vi "PointGrey Grasshopper_Cam.vi"(0 "Operation":T2(ring), 1 "Camera-specific in":variant, 5 "Exposure time (s)":dbl, 7 "Save path":path, 9 "Capture mode":enum16{"Single frame", "Sequence"}(ring), 11 "Capture button":refnum<vi>, 12 "Image in":variant, 14 "Frames in sequence":u32) -> (3 "Camera-specific out":variant, 4 "Status":T1)   [LabVIEW 2018]
uses:
  <vilib>/userdefined/High Color/IMAQdx.ctl
  <vilib>/vision/Image Controls.llb/IMAQ Image.ctl
  <vilib>/vision/driver/IMAQdx.llb/IMAQdx Camera Control Mode.ctl
  <vilib>/vision/driver/IMAQdx.llb/IMAQdx Acquisition Mode.ctl
  <vilib>/Platform/TimedLoop/XDataNode/timing_clust.ctl
  <vilib>/Platform/TimedLoop/XDataNode/nitl_modes.ctl
  <vilib>/Platform/TimedLoop/XDataNode/wakeup.ctl
  <vilib>/vision/driver/IMAQdx.llb/IMAQdx Buffer Number Mode.ctl
  <vilib>/platform/TimedLoop/XDataNode/XDataNode.xnode
  <vilib>/vision/driver/NI_Vision_Acquisition_Software.lvlib
  <resource>/objmgr/imaqdx.rc
  <vilib>/Platform/TimedLoop/XDataNode/XDNodeRunTimeDep.lvlib
  <vilib>/vision/NI_Vision_Development_Module.lvlib
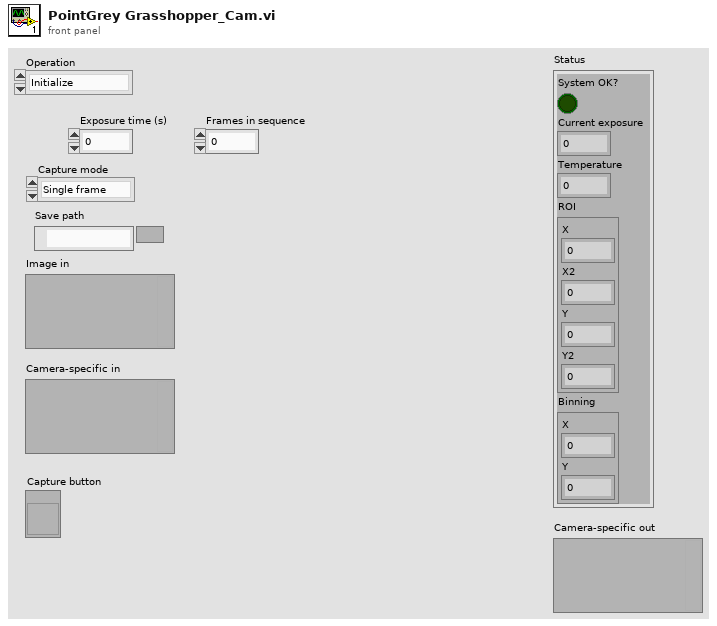
[diagram p1: front panel]
types:
  T1 = cluster{"System OK?":bool, "Current exposure":dbl, "Temperature":dbl, "ROI":cluster{"X":u32, "X2":u32, "Y":u32, "Y2":u32}, "Binning":cluster{"X":u32, "Y":u32}}
  T2 = enum16{"Initialize", "Shut down", "Set capture mode", "Set exposure", "Trigger and read", "Get status", "Other settings"}
  T3 = typedef "IMAQdx.ctl" = refnum<k21>
  T4 = typedef "IMAQ Image.ctl" = refnum<image>
  T5 = typedef "Semaphore RefNum" = refnum<k1>
  T6 = cluster{"Frames to capture":u32, "Current camera":i32, "Camera References":T3[], "Which cameras record":bool[], "Camera event refnums":refnum<event-registration>[], "Image buffers":T4[], "File write access":T5, "Offset and gain":dbl[][], "RGB Channels":enum16{"None", "Camera 1", "Camera 2", "Camera 3"}[], "RGB buffers":T4[], "Camera orientation":enum16{"No rotation, No flip", "No rotation, Flip UD", "No rotation, Flip LR", "Clockwise, No flip", "Clockwise, Flip UD", "Clockwise, Flip LR", "Anticlockwise, No flip", "Anticlockwise, Flip UD", "Anticlockwise, Flip LR"}[]}
  T7 = enum32{"Continuous", "Single frame", "Multi frame"}
  T8 = typedef "NI_Vision_Acquisition_Software.lvlib/IMAQdx Camera Control Mode.ctl" = enum32{"Controller", "Listener"}
  T9 = cluster{"New Image":T4, "Image":refnum<vi>, "FPS target":dbl}
  T10 = enum16{"open", "replace", "create", "open or create", "replace or create", "replace or create with confirmation"}
  T11 = cluster{"File refnum":refnum<file>, "Image File Directory":cluster{cluster{"Field":u16, "Type":u16, "Count":u32, "Value / Offset":u32, "Add IFD Offset?":bool}[], cluster{"Data":u32[], "Add offset?":bool}[]}, "Big endian?":bool, "IFD Offset Size":u32}
  T12 = typedef "NI_Vision_Acquisition_Software.lvlib/IMAQdx Acquisition Mode.ctl" = enum32{"One Shot", "Continuous"}
  T13 = typedef "XDNodeRunTimeDep.lvlib/timing_clust.ctl" = cluster{"Expected End [f-1]":u64, "Actual End [f-1]":u64, "Finished Late? [f-1]":bool, "Expected End [i-1]":u64, "Actual End [i-1]":u64, "Finished Late? [i-1]":bool, "Expected Start [i]":u64, "Actual Start [i]":u64, "Expected Start [f]":u64, "Actual Start [f]":u64, "Source Name":string, "Structure Name":string, "Period":i64, "Deadline":i64, "Offset":i64, "Start":i64, "Priority":i32, "Timeout":i32, "Mode":T14, "Wakeup Reason":T15, "Error":errorcluster, "Source Type":string, "Secondary Source Type":string, "Global End Time":u64, "Global Start Time":u64, "Frame Duration":u64, "Iteration Duration":u64, "Assigned CPU":i32, "I/O Scan Engine Mode":u32}
  T14 = typedef "XDNodeRunTimeDep.lvlib/nitl_modes.ctl" = enum32{"No Change", "Process missed periods, maintain original phase", "Discard missed periods, maintain original phase", "Process missed periods, ignore original phase", "Discard missed periods, ignore original phase"}
  T15 = typedef "XDNodeRunTimeDep.lvlib/wakeup.ctl" = enum32{"Normal", "Aborted", "Asynchronous wakeup", "Timing source error", "Timed loop error", "Timeout"}
  T16 = typedef "NI_Vision_Acquisition_Software.lvlib/IMAQdx Buffer Number Mode.ctl" = enum32{"Next", "Last", "Buffer Number", "Every", "Last New"}
  T17 = typedef "Image Type" = u32
  T18 = enum16{"No rotation, No flip", "No rotation, Flip UD", "No rotation, Flip LR", "Clockwise, No flip", "Clockwise, Flip UD", "Clockwise, Flip LR", "Anticlockwise, No flip", "Anticlockwise, Flip UD", "Anticlockwise, Flip LR"}[]
  T19 = enum16{"None", "Camera 1", "Camera 2", "Camera 3"}[]
  T20 = cluster{"Type":u32, "Version":u32, "Flags":u32, "SerialNumberHigh":u32, "SerialNumberLow":u32, "BusType":u32, "InterfaceName":string, "VendorName":string, "ModelName":string, "CameraFileName":string, "CameraAttributeURL":string}[]
  T21 = enum16{"None", "Camera 1", "Camera 2", "Camera 3"}
  T22 = cluster{"Camera identity":enum16{"Camera 1", "Camera 2", "Camera 3"}, "Timestamp":u64}
  T23 = enum16{"No rotation, No flip", "No rotation, Flip UD", "No rotation, Flip LR", "Clockwise, No flip", "Clockwise, Flip UD", "Clockwise, Flip LR", "Anticlockwise, No flip", "Anticlockwise, Flip UD", "Anticlockwise, Flip LR"}
  T24 = cluster{"element":enum16{"Camera 1", "Camera 2", "Camera 3"}, u64}
  T25 = cluster{"Camera identity":enum16{"Camera 1", "Camera 2", "Camera 3"}, "Timestamp":u64}[]
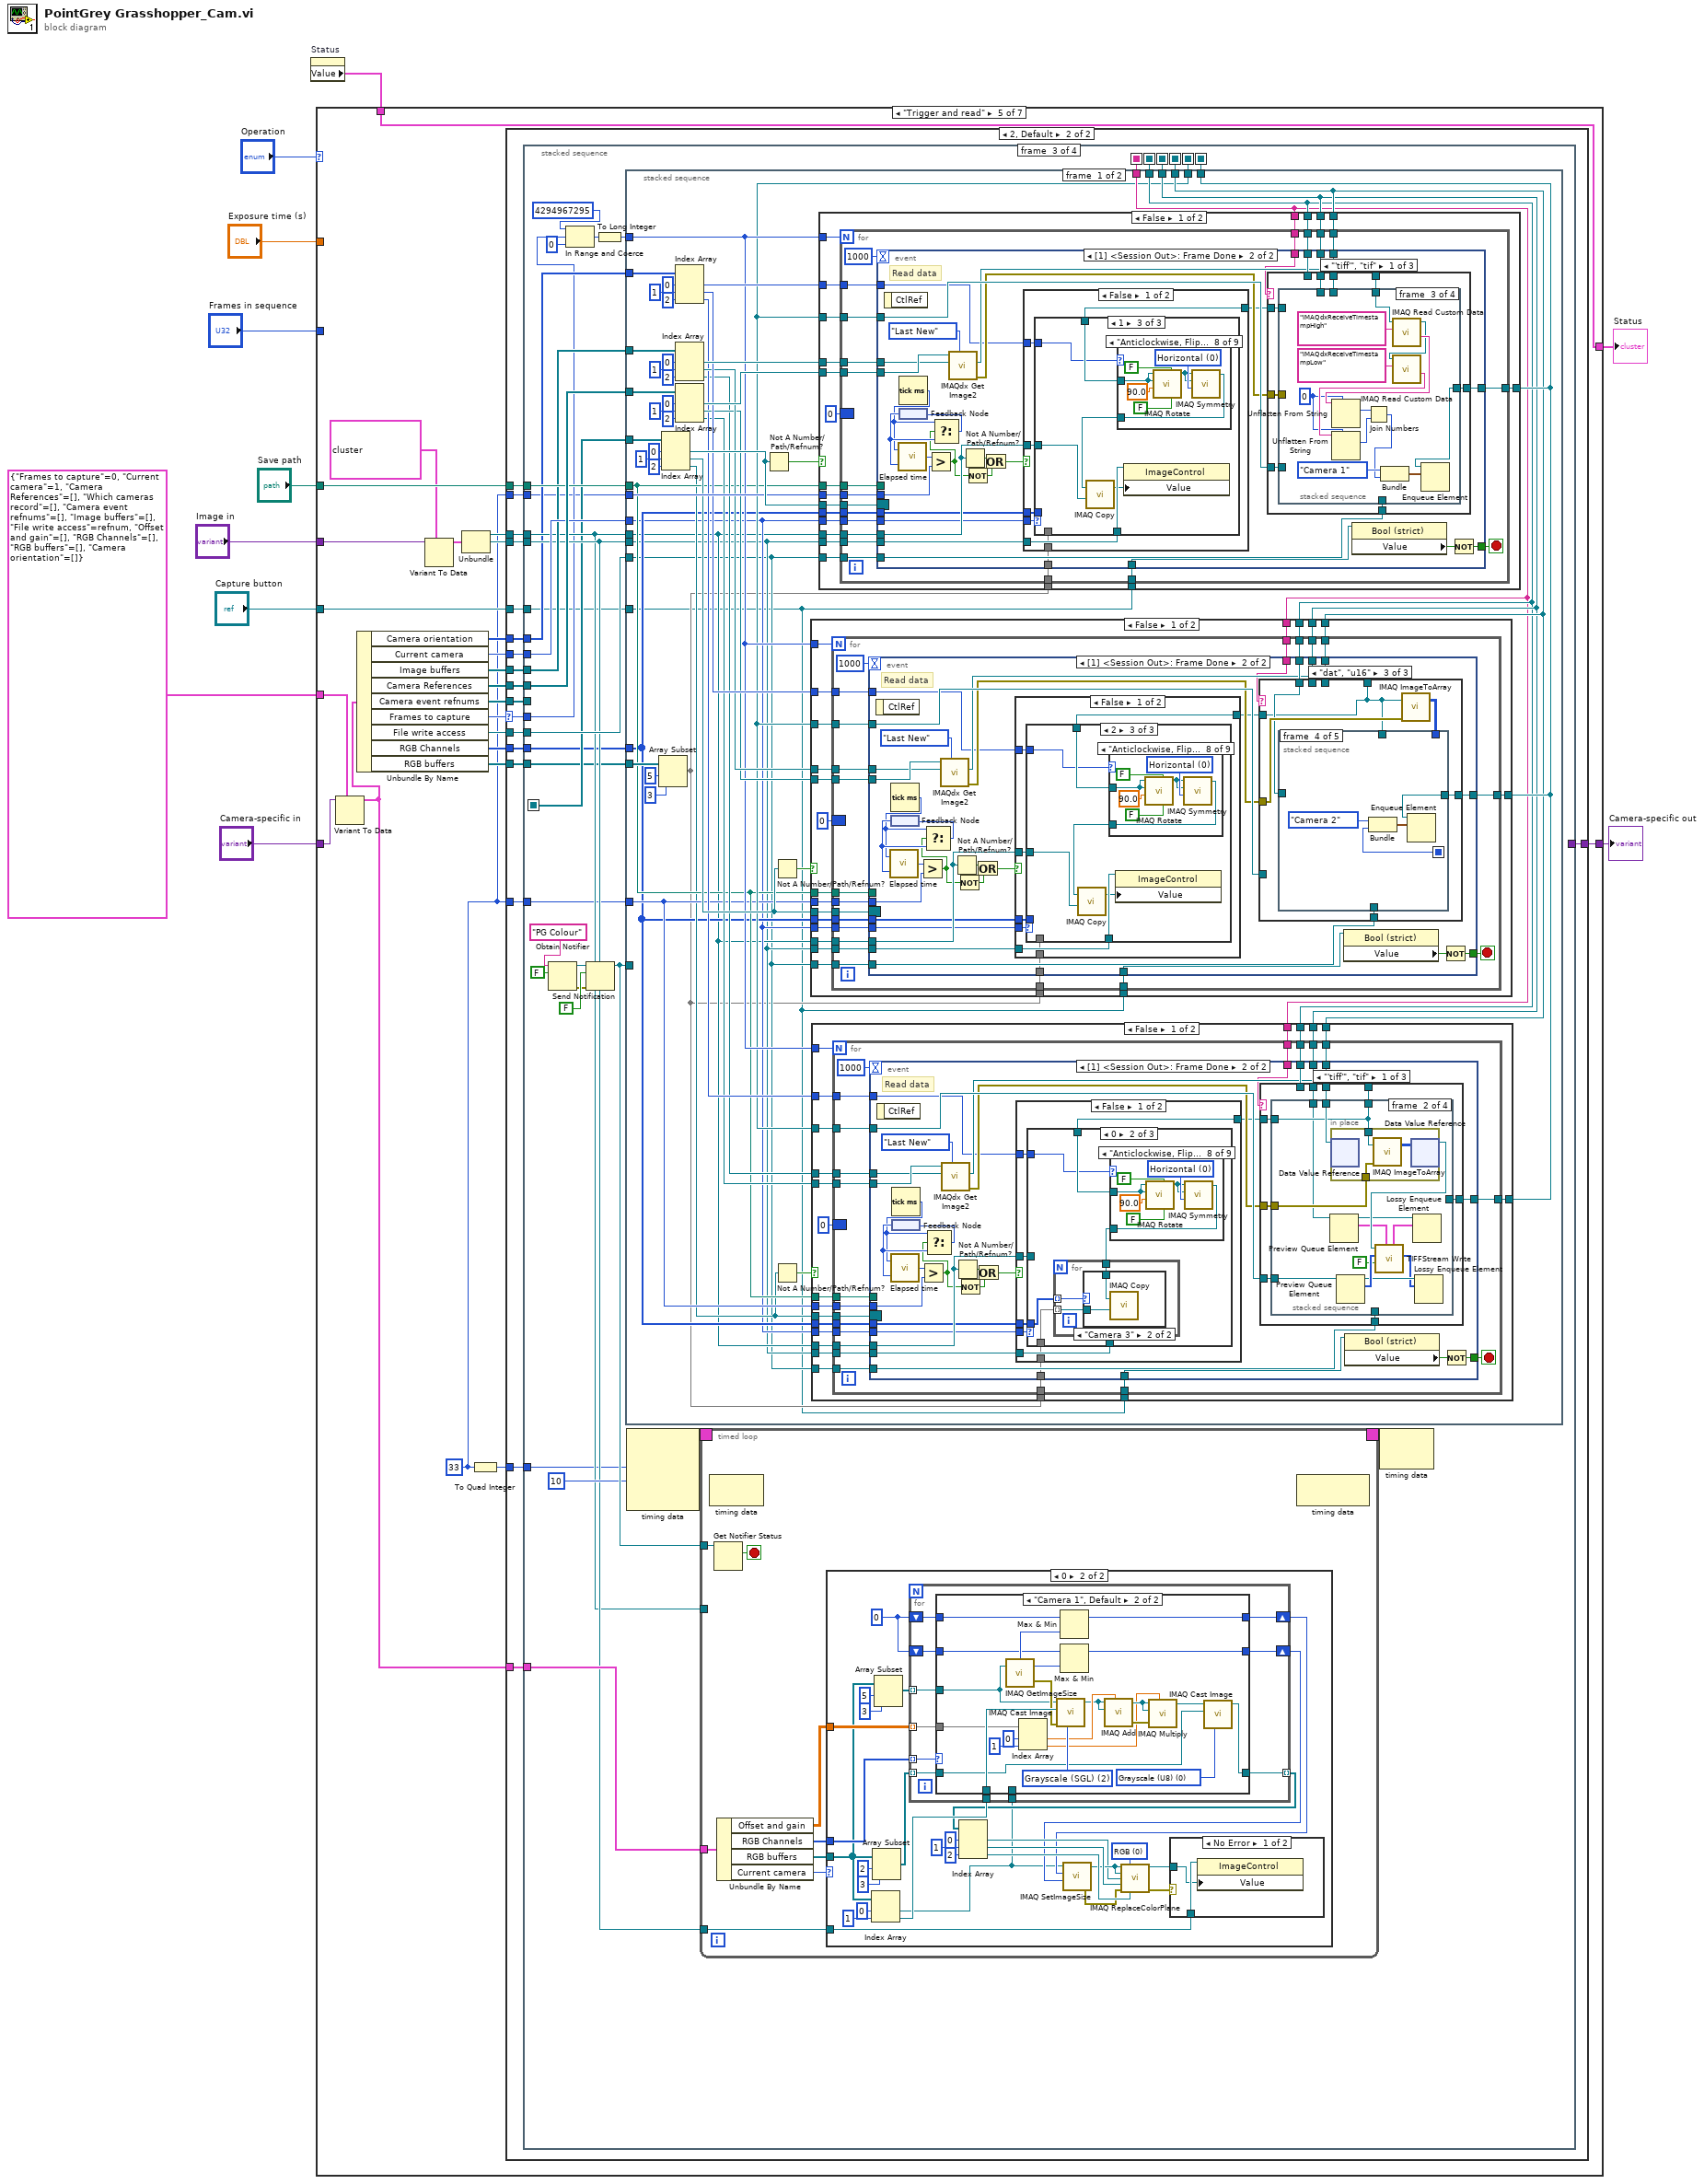
[diagram p0: block diagram]
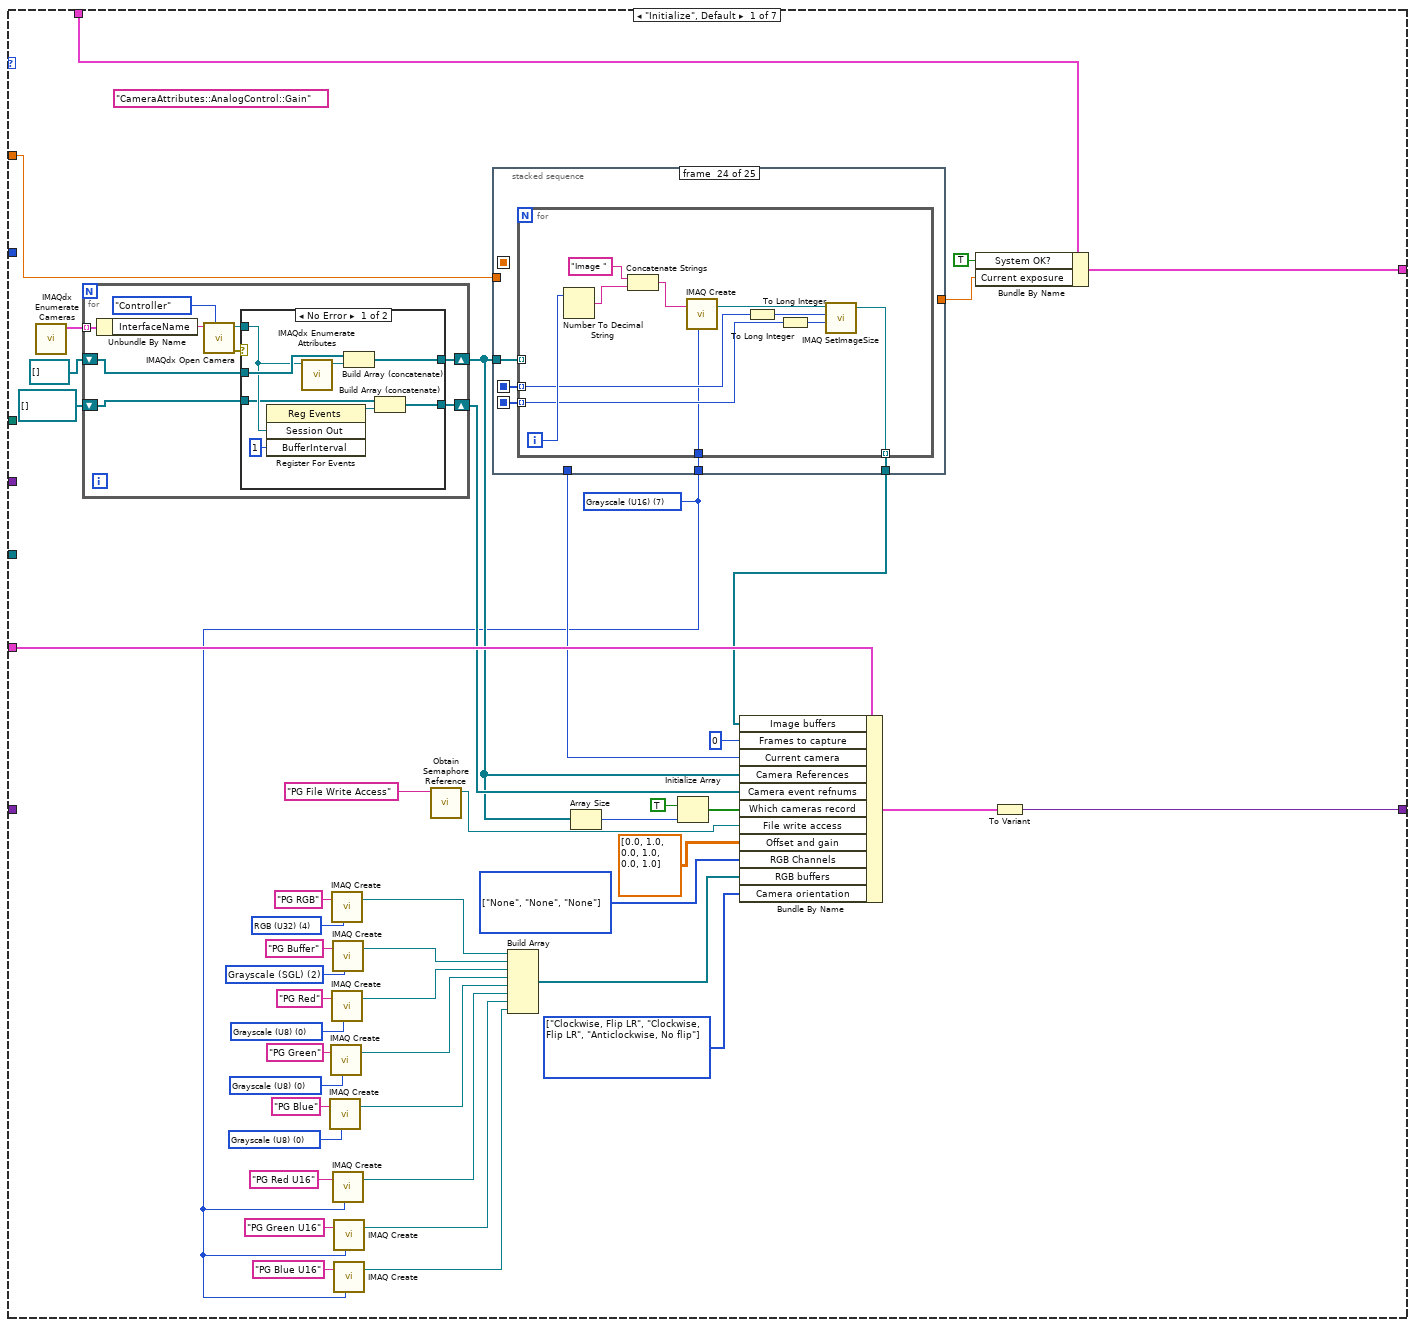
[diagram p2: hidden frame]
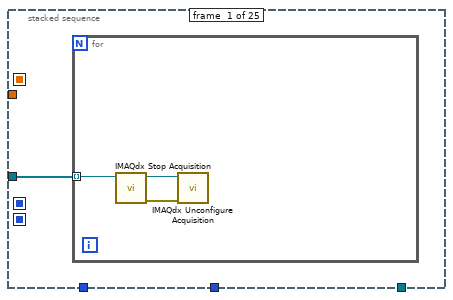
[diagram p3: hidden frame]
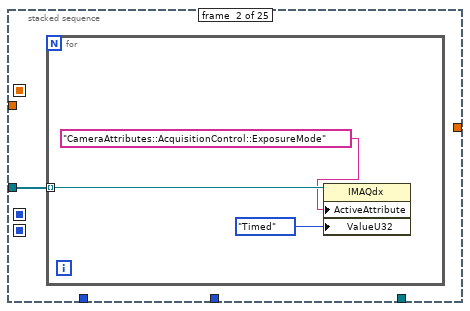
[diagram p4: hidden frame]
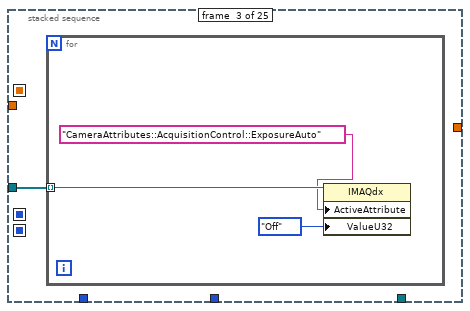
[diagram p5: hidden frame]
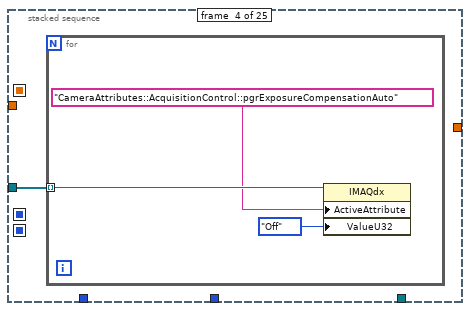
[diagram p6: hidden frame]
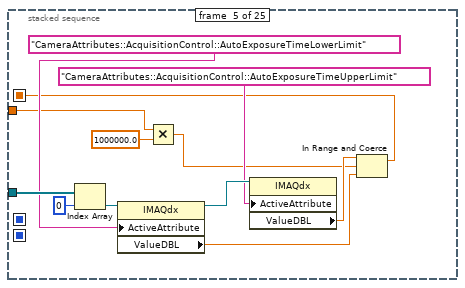
[diagram p7: hidden frame]
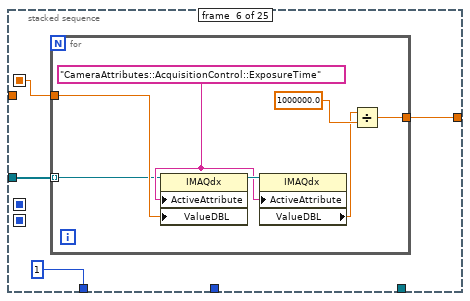
[diagram p8: hidden frame]
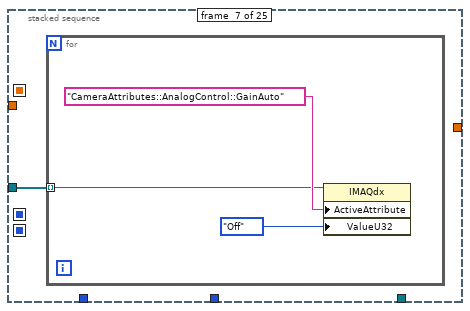
[diagram p9: hidden frame]
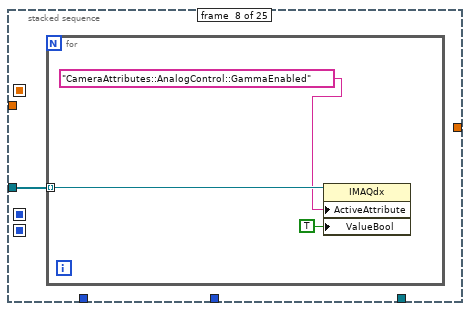
[diagram p10: hidden frame]
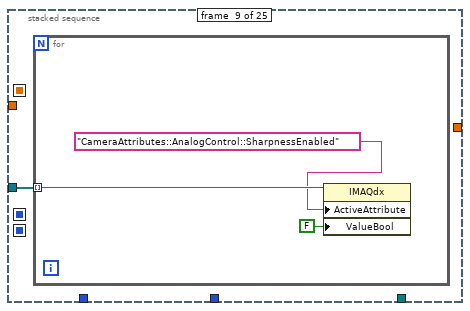
[diagram p11: hidden frame]
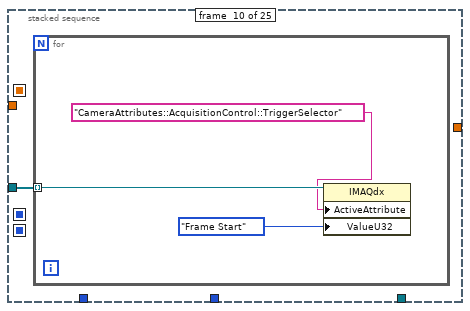
[diagram p12: hidden frame]
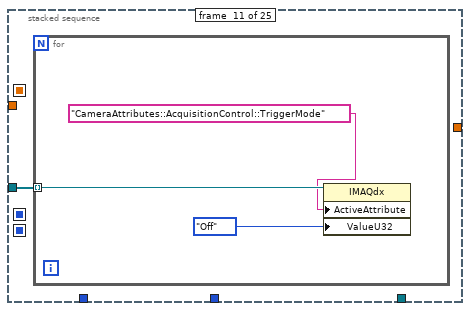
[diagram p13: hidden frame]
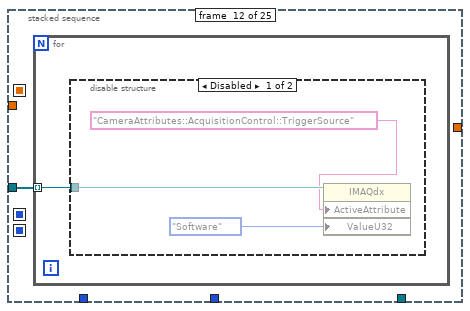
[diagram p14: hidden frame]
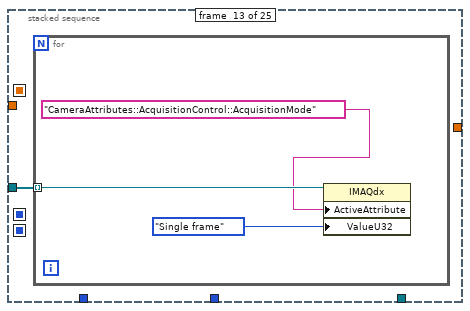
[diagram p16: hidden frame]
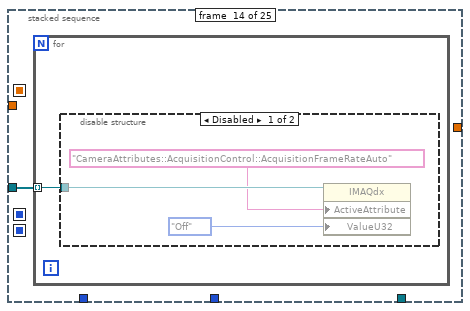
[diagram p17: hidden frame]
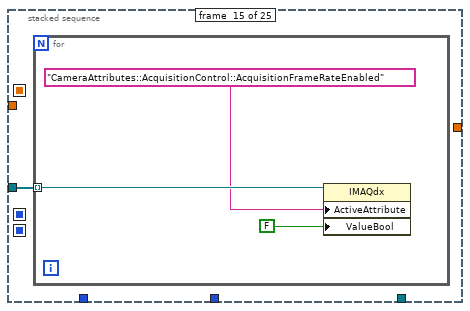
[diagram p19: hidden frame]
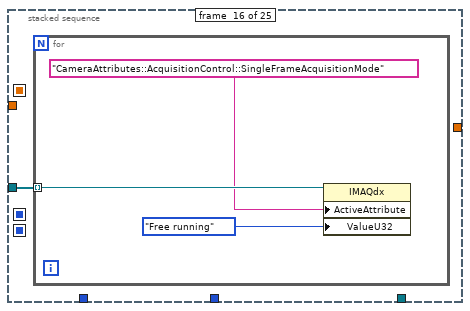
[diagram p20: hidden frame]
diagram:
  n1 = property on="Status" class="Clust (strict)"() -> ("Value"=w9:T1)  [unwired: 2 in, 2 out]
  n2 = case shown="\"Trigger and read\"" "Operation" {
    tunnel: "Exposure time (s)" -> [w47 _ _ w382 _ _ _]
    tunnel: w9 -> [w58 w218 w242 w388 w439 w1774 w1792]
    tunnel: [w57 w218 w242 w387 w439 w1773 w1792] -> w8
    tunnel: "Save path" -> [_ _ _ _ w438 _ _]
    tunnel: "Image in" -> [_ _ _ _ w429 _ _]
    tunnel: [w55 w213 w238 w385 w422 w1770 w1784] -> w5
    tunnel: "Camera-specific in" -> [_ w217 w240 w385 w425 w1770 w1791]
    tunnel: T6 {"Frames to capture"=0, "Current camera"=1, "Camera References"=[], "Which cameras record"=[], "Camera event refnums"=[], "Image buffers"=[], "File write access"=refnum, "Offset and gain"=[], "RGB Channels"=[], "RGB buffers"=[], "Camera orientation"=[]} -> [w56 w212 w239 w386 w437 w1769 w1790]
    tunnel: "Frames in sequence" -> [_ _ w235 _ _ _ _]
    tunnel: "Capture button" -> [_ _ _ _ w421 _ _]
    frame "Initialize", Default {
      w17 = T17 7 items=["Grayscale (U8)", "Grayscale (I16)", "Grayscale (SGL)", "Complex (CSG)", "RGB (U32)", "HSL (U32)", "RGB (U64)", "Grayscale (U16)"] ("Image Type")
      w19 = T18 [enum."Clockwise, Flip LR", enum."Clockwise, Flip LR", enum."Anticlockwise, No flip"] items=["No rotation, No flip", "No rotation, Flip UD", "No rotation, Flip LR", "Clockwise, No flip", "Clockwise, Flip UD", "Clockwise, Flip LR", "Anticlockwise, No flip", "Anticlockwise, Flip UD", "Anticlockwise, Flip LR"] ("Camera orientation")
      w26 = T17 0 items=["Grayscale (U8)", "Grayscale (I16)", "Grayscale (SGL)", "Complex (CSG)", "RGB (U32)", "HSL (U32)", "RGB (U64)", "Grayscale (U16)"] ("Image Type")
      w27 = T17 0 items=["Grayscale (U8)", "Grayscale (I16)", "Grayscale (SGL)", "Complex (CSG)", "RGB (U32)", "HSL (U32)", "RGB (U64)", "Grayscale (U16)"] ("Image Type")
      w28 = T17 0 items=["Grayscale (U8)", "Grayscale (I16)", "Grayscale (SGL)", "Complex (CSG)", "RGB (U32)", "HSL (U32)", "RGB (U64)", "Grayscale (U16)"] ("Image Type")
      w29 = T17 2 items=["Grayscale (U8)", "Grayscale (I16)", "Grayscale (SGL)", "Complex (CSG)", "RGB (U32)", "HSL (U32)", "RGB (U64)", "Grayscale (U16)"] ("Image Type")
      w30 = T17 4 items=["Grayscale (U8)", "Grayscale (I16)", "Grayscale (SGL)", "Complex (CSG)", "RGB (U32)", "HSL (U32)", "RGB (U64)", "Grayscale (U16)"] ("Image Type")
      w36 = T19 [enum."None", enum."None", enum."None"] items=["None", "Camera 1", "Camera 2", "Camera 3"] ("RGB Channels")
      (unwired) "CameraAttributes::AnalogControl::Gain"
      n3 = call <vilib>:"IMAQdx Enumerate Cameras.vi"() -> ("Camera Information Array"=w53:T20)  [unwired: 10 in, 1 out]
      n4 = for {
        tunnel: w53 -> [w198] mode=indexing
        shift-right: [w193] -> w45
        shift-left: T3[] [] -> [w191]
        shift-right: [w194] -> w50
        shift-left: refnum<event-registration>[] [] -> [w190]
        n5 = Unbundle By Name(w198) -> ("InterfaceName"=w197:string)
        n6 = call <vilib>:"IMAQdx Open Camera.vi"("Camera Control Mode"=IMAQdx_Camera_Control_Mode."Controller", "Session In"=w197) -> ("error out"=w192:errorcluster, "Session Out"=w195:T3)  [unwired: 8 in]
        n7 = case shown="No Error" w192 {
          tunnel: w195 -> [w202 _]
          tunnel: [w201 w207] -> w194
          tunnel: [w204 w208] -> w193
          tunnel: w191 -> [w203 w208]
          tunnel: w190 -> [w199 w207]
          frame No Error {
            n8 = register-events(w202, u32 1 ("BufferInterval")) -> (reference out=w200:refnum<event-registration>)  [unwired: 2 in, 1 out]
            n9 = call <vilib>:"IMAQdx Enumerate Attributes.vi"("Session In"=w202) -> ("Session Out"=w205:T3)  [unwired: 8 in, 2 out]
            n10 = Build Array (concatenate)(w203, w205) -> (w204:T3[])
            n11 = Build Array (concatenate)(w199, w200) -> (w201:refnum<event-registration>[])
          }
          frame Error {
          }
        }
      }
      n12 = call "IMAQ Create"("Image Name"="PG Blue", "Image Type"=w26) -> ("New Image"=w21:T4)  [unwired: 3 in, 1 out]
      n13 = call "IMAQ Create"("Image Name"="PG Green", "Image Type"=w27) -> ("New Image"=w22:T4)  [unwired: 3 in, 1 out]
      n14 = call "IMAQ Create"("Image Name"="PG RGB", "Image Type"=w30) -> ("New Image"=w25:T4)  [unwired: 3 in, 1 out]
      n15 = call "IMAQ Create"("Image Name"="PG Red", "Image Type"=w28) -> ("New Image"=w23:T4)  [unwired: 3 in, 1 out]
      n16 = call "IMAQ Create"("Image Name"="PG Buffer", "Image Type"=w29) -> ("New Image"=w24:T4)  [unwired: 3 in, 1 out]
      n17 = call "IMAQ Create"("Image Name"="PG Red U16", "Image Type"=w17) -> ("New Image"=w16:T4)  [unwired: 3 in, 1 out]
      n18 = call "IMAQ Create"("Image Name"="PG Green U16", "Image Type"=w17) -> ("New Image"=w14:T4)  [unwired: 3 in, 1 out]
      n19 = call "IMAQ Create"("Image Name"="PG Blue U16", "Image Type"=w17) -> ("New Image"=w15:T4)  [unwired: 3 in, 1 out]
      n20 = call <vilib>:"Obtain Semaphore Reference.vi"("name (unnamed)"="PG File Write Access") -> ("semaphore"=w38:T5)  [unwired: 4 in, 2 out]
      n21 = stacked-sequence {
        seq-local: [_ _ _ _ w78 _ _ _ _ _ _ _ _ _ _ _ _ _ _ _ _ _ _ _ _] -> [_ _ _ _ _ w87 _ _ _ _ _ _ _ _ _ _ _ _ _ _ _ _ _ _ _]
        seq-local: [_ _ _ _ _ _ _ _ _ _ _ _ _ _ _ _ _ w144 _ _ _ _ _ _ _] -> [_ _ _ _ _ _ _ _ _ _ _ _ _ _ _ _ _ _ _ _ _ _ _ w175 _]
        seq-local: [_ _ _ _ _ _ _ _ _ _ _ _ _ _ _ _ _ _ w150 _ _ _ _ _ _] -> [_ _ _ _ _ _ _ _ _ _ _ _ _ _ _ _ _ _ _ _ _ _ _ w174 _]
        tunnel: w45 -> [w59 w63 w67 w71 w84 w90 w98 w102 w106 w110 w114 w118 w123 w127 w132 w136 w140 w145 w151 w156 w160 w164 w168 w176 w188]
        tunnel: [_ _ _ _ _ 1 ("index") _ _ _ _ _ _ _ _ _ _ _ _ _ _ _ _ _ _ _] -> w48
        tunnel: w47 -> [_ _ _ _ w76 _ _ _ _ _ _ _ _ _ _ _ _ _ _ _ _ _ _ _ _]
        tunnel: [_ _ _ _ _ w88 _ _ _ _ _ _ _ _ _ _ _ _ _ _ _ _ _ _ _] -> w46
        tunnel: [_ _ _ _ _ _ _ _ _ _ _ _ _ _ _ _ _ _ _ _ _ _ _ w173 _] -> w41
        tunnel: w17 -> [_ _ _ _ _ _ _ _ _ _ _ _ _ _ _ _ _ _ _ _ _ _ _ w172 _]
        frame #0 {
          n22 = for {
            tunnel: w59 -> [w62] mode=indexing
            n23 = call <vilib>:"IMAQdx Stop Acquisition.vi"("Session In"=w62) -> ("error out"=w60:errorcluster, "Session Out"=w61:T3)  [unwired: 9 in]
            n24 = call <vilib>:"IMAQdx Unconfigure Acquisition.vi"("error in"=w60, "Session In"=w61) -> ()  [unwired: 8 in, 2 out]
          }
        }
        frame #1 {
          n25 = for {
            tunnel: w63 -> [w66] mode=indexing
            n26 = property class="IMAQdx"(reference=w66, "ActiveAttribute"="CameraAttributes::AcquisitionControl::ExposureMode", "ValueU32"=enum32{"Timed", "Trigger Width"}."Timed") -> ()  [unwired: 1 in, 2 out]
          }
        }
        frame #2 {
          n27 = for {
            tunnel: w67 -> [w70] mode=indexing
            n28 = property class="IMAQdx"(reference=w70, "ActiveAttribute"="CameraAttributes::AcquisitionControl::ExposureAuto", "ValueU32"=enum32{"Off", "Once", "Continuous"}."Off") -> ()  [unwired: 1 in, 2 out]
          }
        }
        frame #3 {
          n29 = for {
            tunnel: w71 -> [w74] mode=indexing
            n30 = property class="IMAQdx"(reference=w74, "ActiveAttribute"="CameraAttributes::AcquisitionControl::pgrExposureCompensationAuto", "ValueU32"=enum32{"Off", "Once", "Continuous"}."Off") -> ()  [unwired: 1 in, 2 out]
          }
        }
        frame #4 {
          n31 = Index Array(array=w84, index=0) -> (element=w86:T3)
          n32 = property class="IMAQdx"(reference=w86, "ActiveAttribute"="CameraAttributes::AcquisitionControl::AutoExposureTimeLowerLimit") -> (reference out=w82:T3, "ValueDBL"=w80:dbl)  [unwired: 1 in, 1 out]
          n33 = Multiply(x=w76, y=1000000.0) -> (x*y=w75:dbl)
          n34 = property class="IMAQdx"(reference=w82, "ActiveAttribute"="CameraAttributes::AcquisitionControl::AutoExposureTimeUpperLimit") -> ("ValueDBL"=w79:dbl)  [unwired: 1 in, 2 out]
          n35 = In Range and Coerce(upper limit=w79, x=w75, lower limit=w80) -> (coerced(x)=w78:dbl)  [unwired: 1 out]
        }
        frame #5 {
          n36 = for {
            tunnel: w90 -> [w91] mode=indexing
            tunnel: [w94] -> w88
            tunnel: w87 -> [w92]
            w93 = "CameraAttributes::AcquisitionControl::ExposureTime"
            n37 = property class="IMAQdx"(reference=w91, "ActiveAttribute"=w93, "ValueDBL"=w92) -> (reference out=w97:T3)  [unwired: 1 in, 1 out]
            n38 = property class="IMAQdx"(reference=w97, "ActiveAttribute"=w93) -> ("ValueDBL"=w95:dbl)  [unwired: 1 in, 2 out]
            n39 = Divide(x=w95, y=1000000.0) -> (x/y=w94:dbl)
          }
        }
        frame #6 {
          n40 = for {
            tunnel: w98 -> [w99] mode=indexing
            n41 = property class="IMAQdx"(reference=w99, "ActiveAttribute"="CameraAttributes::AnalogControl::GainAuto", "ValueU32"=enum32{"Off", "Once", "Continuous"}."Off") -> ()  [unwired: 1 in, 2 out]
          }
        }
        frame #7 {
          n42 = for {
            tunnel: w102 -> [w105] mode=indexing
            n43 = property class="IMAQdx"(reference=w105, "ActiveAttribute"="CameraAttributes::AnalogControl::GammaEnabled", "ValueBool"=TRUE) -> ()  [unwired: 1 in, 2 out]
          }
        }
        frame #8 {
          n44 = for {
            tunnel: w106 -> [w109] mode=indexing
            n45 = property class="IMAQdx"(reference=w109, "ActiveAttribute"="CameraAttributes::AnalogControl::SharpnessEnabled", "ValueBool"=FALSE) -> ()  [unwired: 1 in, 2 out]
          }
        }
        frame #9 {
          n46 = for {
            tunnel: w110 -> [w113] mode=indexing
            n47 = property class="IMAQdx"(reference=w113, "ActiveAttribute"="CameraAttributes::AcquisitionControl::TriggerSelector", "ValueU32"=enum32{"Frame Start", "Exposure Active"}."Frame Start") -> ()  [unwired: 1 in, 2 out]
          }
        }
        frame #10 {
          n48 = for {
            tunnel: w114 -> [w117] mode=indexing
            n49 = property class="IMAQdx"(reference=w117, "ActiveAttribute"="CameraAttributes::AcquisitionControl::TriggerMode", "ValueU32"=enum32{"Off", "On"}."Off") -> ()  [unwired: 1 in, 2 out]
          }
        }
        frame #11 {
          n50 = for {
            tunnel: w118 -> [w119] mode=indexing
            n51 = disable-structure shown="Disabled" {
              disable-tunnel: w119 -> [w122 _]
              frame Disabled {
                n52 = property class="IMAQdx"(reference=w122, "ActiveAttribute"="CameraAttributes::AcquisitionControl::TriggerSource", "ValueU32"=enum32{"Software", "Line 0", "Line 2", "Line 3"}."Software") -> ()  [unwired: 1 in, 2 out]
              }
              frame Enabled {
              }
            }
          }
        }
        frame #12 {
          n53 = for {
            tunnel: w123 -> [w126] mode=indexing
            n54 = property class="IMAQdx"(reference=w126, "ActiveAttribute"="CameraAttributes::AcquisitionControl::AcquisitionMode", "ValueU32"=T7."Single frame") -> ()  [unwired: 1 in, 2 out]
          }
        }
        frame #13 {
          n55 = for {
            tunnel: w127 -> [w128] mode=indexing
            n56 = disable-structure shown="Disabled" {
              disable-tunnel: w128 -> [w131 _]
              frame Disabled {
                n57 = property class="IMAQdx"(reference=w131, "ActiveAttribute"="CameraAttributes::AcquisitionControl::AcquisitionFrameRateAuto", "ValueU32"=enum32{"Off", "Continuous"}."Off") -> ()  [unwired: 1 in, 2 out]
              }
              frame Enabled {
              }
            }
          }
        }
        frame #14 {
          n58 = for {
            tunnel: w132 -> [w135] mode=indexing
            n59 = property class="IMAQdx"(reference=w135, "ActiveAttribute"="CameraAttributes::AcquisitionControl::AcquisitionFrameRateEnabled", "ValueBool"=FALSE) -> ()  [unwired: 1 in, 2 out]
          }
        }
        frame #15 {
          n60 = for {
            tunnel: w136 -> [w139] mode=indexing
            n61 = property class="IMAQdx"(reference=w139, "ActiveAttribute"="CameraAttributes::AcquisitionControl::SingleFrameAcquisitionMode", "ValueU32"=enum16{"Free running", "Triggered"}."Free running") -> ()  [unwired: 1 in, 2 out]
          }
        }
        frame #16 {
          n62 = for {
            tunnel: w140 -> [w143] mode=indexing
            w142 = u32 17563654 items=["Mono 8"=17301505, "Mono 12 Packed (IIDC-msb)"=17563654, "Mono 12 Packed"=17563719, "Mono 16"=17825799]
            n63 = property class="IMAQdx"(reference=w143, "ActiveAttribute"="CameraAttributes::ImageFormatControl::PixelFormat", "ValueU32"=w142) -> ()  [unwired: 1 in, 2 out]
          }
        }
        frame #17 {
          n64 = for {
            tunnel: w145 -> [w149] mode=indexing
            tunnel: [w146] -> w144 mode=indexing
            w148 = "CameraAttributes::ImageFormatControl::Width"
            n65 = property class="IMAQdx"(reference=w149, "ActiveAttribute"=w148) -> (reference out=w147:T3, "MaxU32"=w146:u32)  [unwired: 1 in, 1 out]
            n66 = property class="IMAQdx"(reference=w147, "ActiveAttribute"=w148, "ValueU32"=w146) -> ()  [unwired: 1 in, 2 out]
          }
        }
        frame #18 {
          n67 = for {
            tunnel: w151 -> [w155] mode=indexing
            tunnel: [w152] -> w150 mode=indexing
            w154 = "CameraAttributes::ImageFormatControl::Height"
            n68 = property class="IMAQdx"(reference=w155, "ActiveAttribute"=w154) -> (reference out=w153:T3, "MaxU32"=w152:u32)  [unwired: 1 in, 1 out]
            n69 = property class="IMAQdx"(reference=w153, "ActiveAttribute"=w154, "ValueU32"=w152) -> ()  [unwired: 1 in, 2 out]
          }
        }
        frame #19 {
          n70 = for {
            tunnel: w156 -> [w158] mode=indexing
            n71 = property class="IMAQdx"(reference=w158, "ActiveAttribute"="CameraAttributes::ImageFormatControl::OffsetX", "ValueU32"=u32 0) -> ()  [unwired: 1 in, 2 out]
          }
        }
        frame #20 {
          n72 = for {
            tunnel: w160 -> [w162] mode=indexing
            n73 = property class="IMAQdx"(reference=w162, "ActiveAttribute"="CameraAttributes::ImageFormatControl::OffsetY", "ValueU32"=u32 0) -> ()  [unwired: 1 in, 2 out]
          }
        }
        frame #21 {
          n74 = for {
            tunnel: w164 -> [w166] mode=indexing
            n75 = property class="IMAQdx"(reference=w166, "ActiveAttribute"="CameraAttributes::ImageFormatControl::BinningVertical", "ValueU32"=u32 1) -> ()  [unwired: 1 in, 2 out]
          }
        }
        frame #22 {
          n76 = for {
            tunnel: w168 -> [w170] mode=indexing
            w169 = u16 7 items=["Standard"=0, "2x2 Binning"=1, "2x2 Decimation"=2, "High sensitivity 12-bit ADC"=7]
            n77 = property class="IMAQdx"(reference=w170, "ActiveAttribute"="CameraAttributes::ImageFormatControl::VideoMode", "ValueU32"=w169) -> ()  [unwired: 1 in, 2 out]
          }
        }
        frame #23 {
          n78 = for {
            tunnel: w176 -> [_] mode=indexing
            tunnel: w175 -> [w181] mode=indexing
            tunnel: w174 -> [w180] mode=indexing
            tunnel: [w182] -> w173 mode=indexing
            tunnel: w172 -> [w177]
            i -> [w186]
            n79 = Number To Decimal String(number=w186) -> (decimal integer string=w185:string)  [unwired: 1 in]
            n80 = Concatenate Strings("Image ", w185) -> (w184:string)
            n81 = call "IMAQ Create"("Image Name"=w184, "Image Type"=w177) -> ("New Image"=w183:T4)  [unwired: 3 in, 1 out]
            n82 = To Long Integer(number=w181) -> (32bit integer=w179:i32)
            n83 = To Long Integer(number=w180) -> (32bit integer=w178:i32)
            n84 = call "IMAQ SetImageSize"("Y Resolution"=w178, "X Resolution"=w179, "Image"=w183) -> ("Image Out"=w182:T4)  [unwired: 2 in, 1 out]
          }
        }
        frame #24 {
          n85 = for {
            tunnel: w188 -> [w189] mode=indexing
            n86 = call <vilib>:"IMAQdx Configure Grab.vi"("Session In"=w189) -> ()  [unwired: 9 in, 2 out]
          }
        }
      }
      n87 = Build Array(w25, w24, w23, w22, w21, w16, w14, w15) -> (w20:T4[])
      n88 = Array Size(array=w45) -> (size(s)=w43:i32)
      n89 = Initialize Array(TRUE, w43) -> (w42:bool[])
      n90 = Bundle By Name(cluster=w56, "Image buffers"=w41, "Frames to capture"=u32 0, "Current camera"=w48, "Camera References"=w45, "Camera event refnums"=w50, "Which cameras record"=w42, "File write access"=w38, "Offset and gain"=dbl[][] [[0.0, 1.0], [0.0, 1.0], [0.0, 1.0]], "RGB Channels"=w36, "RGB buffers"=w20, "Camera orientation"=w19) -> (w51:T6)
      n91 = Bundle By Name(cluster=w58, "System OK?"=TRUE, "Current exposure"=w46) -> (w57:T1)
      n92 = To Variant(anything=w51) -> (Variant=w55:variant)
    }
    frame "Shut down" {
      n93 = Variant To Data(type=w212, Variant=w217) -> (data=w216:T6)  [unwired: 1 in, 1 out]
      n94 = Unbundle By Name(w216) -> ("Camera References"=w215:T3[], "Camera event refnums"=w214:refnum<event-registration>[], "File write access"=w211:T5, "Image buffers"=w210:T4[], "RGB buffers"=w209:T4[])
      n95 = for {
        tunnel: w210 -> [w220] mode=indexing
        n96 = call "IMAQ Dispose"("Image"=w220) -> ()  [unwired: 5 in, 1 out]
      }
      n97 = for {
        tunnel: w209 -> [w219] mode=indexing
        n98 = call "IMAQ Dispose"("Image"=w219) -> ()  [unwired: 5 in, 1 out]
      }
      n99 = stacked-sequence {
        tunnel: w215 -> [w221 _]
        tunnel: w214 -> [_ w227]
        frame #0 {
          n100 = for {
            tunnel: w221 -> [w222] mode=indexing
            n101 = call <vilib>:"IMAQdx Stop Acquisition.vi"("Session In"=w222) -> ("error out"=w226:errorcluster, "Session Out"=w225:T3)  [unwired: 9 in]
            n102 = call <vilib>:"IMAQdx Unconfigure Acquisition.vi"("error in"=w226, "Session In"=w225) -> ("error out"=w224:errorcluster, "Session Out"=w223:T3)  [unwired: 8 in]
            n103 = call <vilib>:"IMAQdx Close Camera.vi"("error in"=w224, "Session In"=w223) -> ()  [unwired: 9 in, 1 out]
          }
        }
        frame #1 {
          n104 = for {
            tunnel: w227 -> [w229] mode=indexing
            n105 = Unregister For Events(event registration refnum=w229) -> (error out=w228:errorcluster)  [unwired: 1 in]
            n106 = call <vilib>:"Clear Errors.vi"("error in (no error)"=w228) -> ()  [unwired: 5 in, 2 out]
          }
        }
      }
      n107 = call <vilib>:"Release Semaphore Reference.vi"("semaphore"=w211) -> ()  [unwired: 9 in, 2 out]
      n108 = To Variant(anything=w212) -> (Variant=w213:variant)
    }
    frame "Set capture mode" {
      n109 = Variant To Data(type=w239, Variant=w240) -> (data=w234:T6)  [unwired: 1 in, 1 out]
      n110 = Unbundle By Name(w234) -> ("Camera References"=w233:T3[], "Camera event refnums"=w231:refnum<event-registration>[], "Which cameras record"=w232:bool[])
      n111 = case shown="\"Sequence\"" "Capture mode" {
        tunnel: [w243 w313] -> w236
        tunnel: w235 -> [w244 w314]
        tunnel: w233 -> [w248 w318]
        tunnel: w232 -> [w247 w317]
        tunnel: w231 -> [w246 w316]
        tunnel: [w245 w315] -> w230
        frame "Sequence" {
          n112 = stacked-sequence {
            tunnel: w248 -> [_ w257]
            tunnel: w247 -> [_ w256]
            tunnel: w246 -> [w250 w253]
            tunnel: [_ w255] -> w245
            tunnel: w244 -> [w249 w254]
            tunnel: [w249 _] -> w243
            frame #0 {
              n113 = disable-structure shown="Enabled" {
                disable-tunnel: w250 -> [w251 _]
                frame Disabled {
                  n114 = for {
                    tunnel: w251 -> [w252] mode=indexing
                    n115 = Unregister For Events(event registration refnum=w252) -> ()  [unwired: 1 in, 1 out]
                  }
                }
                frame Enabled {
                }
              }
            }
            frame #1 {
              n116 = for {
                tunnel: w257 -> [w262] mode=indexing
                tunnel: w256 -> [w263] mode=indexing
                shift-right: [w261] -> w255
                shift-left: w253 -> [w260]
                tunnel: w254 -> [w259]
                i -> [w258]
                n117 = case shown="True" w263 {
                  tunnel: w262 -> [_ w267]
                  tunnel: [w264 w268] -> w261
                  tunnel: w260 -> [w264 w269]
                  tunnel: w259 -> [_ w266]
                  tunnel: w258 -> [_ w265]
                  frame False {
                  }
                  frame True {
                    n118 = stacked-sequence {
                      tunnel: w269 -> [_ _ _ _ _ _ _ _ w300 _]
                      tunnel: [_ _ _ _ _ _ _ _ w301 _] -> w268
                      tunnel: w267 -> [w272 w273 w281 w285 w288 w292 w294 w297 w302 w310]
                      tunnel: w266 -> [_ _ w280 _ _ _ _ _ _ _]
                      tunnel: w265 -> [_ _ _ _ _ _ _ _ w299 _]
                      frame #0 {
                        n119 = call <vilib>:"IMAQdx Stop Acquisition.vi"("Session In"=w272) -> ("error out"=w270:errorcluster, "Session Out"=w271:T3)  [unwired: 9 in]
                        n120 = call <vilib>:"IMAQdx Unconfigure Acquisition.vi"("error in"=w270, "Session In"=w271) -> ()  [unwired: 8 in, 2 out]
                      }
                      frame #1 {
                        n121 = disable-structure shown="Enabled" {
                          disable-tunnel: w273 -> [w274 w277]
                          frame Disabled {
                            n122 = property class="IMAQdx"(reference=w274, "ActiveAttribute"="CameraAttributes::AcquisitionControl::AcquisitionMode", "ValueU32"=T7."Multi frame") -> ()  [unwired: 1 in, 2 out]
                          }
                          frame Enabled {
                            n123 = property class="IMAQdx"(reference=w277, "ActiveAttribute"="CameraAttributes::AcquisitionControl::AcquisitionMode", "ValueU32"=T7."Continuous") -> ()  [unwired: 1 in, 2 out]
                          }
                        }
                      }
                      frame #2 {
                        n124 = disable-structure shown="Enabled" {
                          disable-tunnel: w281 -> [w283 _]
                          disable-tunnel: w280 -> [w282 _]
                          frame Disabled {
                            n125 = property class="IMAQdx"(reference=w283, "ActiveAttribute"="CameraAttributes::AcquisitionControl::AcquisitionFrameCount", "ValueU32"=w282) -> ()  [unwired: 1 in, 2 out]
                          }
                          frame Enabled {
                          }
                        }
                      }
                      frame #3 {
                        n126 = property class="IMAQdx"(reference=w285, "ActiveAttribute"="CameraAttributes::AcquisitionControl::TriggerSource", "ValueU32"=enum32{"Software", "Line 0", "Line 2", "Line 3"}."Software") -> ()  [unwired: 1 in, 2 out]
                      }
                      frame #4 {
                        n127 = property class="IMAQdx"(reference=w288, "ActiveAttribute"="CameraAttributes::AcquisitionControl::TriggerSelector", "ValueU32"=enum32{"Frame Start", "Exposure Active"}."Frame Start") -> ()  [unwired: 1 in, 2 out]
                      }
                      frame #5 {
                        n128 = property class="IMAQdx"(reference=w292, "ActiveAttribute"="CameraAttributes::AcquisitionControl::TriggerMode", "ValueU32"=enum32{"Off", "On"}."Off") -> ()  [unwired: 1 in, 2 out]
                      }
                      frame #6 {
                        n129 = property class="IMAQdx"(reference=w294, "ActiveAttribute"="CameraAttributes::AcquisitionControl::SingleFrameAcquisitionMode", "ValueU32"=enum16{"Free running", "Triggered"}."Triggered") -> ()  [unwired: 1 in, 2 out]
                      }
                      frame #7 {
                        n130 = disable-structure shown="Enabled" {
                          disable-tunnel: w297 -> [w298 _]
                          frame Disabled {
                            n131 = call <vilib>:"IMAQdx Configure Grab.vi"("Session In"=w298) -> ()  [unwired: 9 in, 2 out]
                          }
                          frame Enabled {
                          }
                        }
                      }
                      frame #8 {
                        n132 = disable-structure shown="Enabled" {
                          disable-tunnel: w302 -> [w308 _]
                          disable-tunnel: [w306 w309] -> w301
                          disable-tunnel: w300 -> [w305 w309]
                          disable-tunnel: w299 -> [w303 _]
                          frame Disabled {
                            n133 = register-events(w308, u32 1 ("BufferInterval")) -> (reference out=w304:refnum<event-registration>)  [unwired: 2 in, 1 out]
                            n134 = Replace Array Subset(array=w305, new element=w304, index=w303) -> (w306:refnum<event-registration>[])
                          }
                          frame Enabled {
                          }
                        }
                      }
                      frame #9 {
                        n135 = property class="IMAQdx"(reference=w310, "ActiveAttribute"="AcquisitionAttributes::ReceiveTimestampMode", "ValueU32"=enum16{"None", "Tick count", "System time"}."System time") -> ()  [unwired: 1 in, 2 out]
                      }
                    }
                  }
                }
              }
            }
          }
        }
        frame "Single frame", Default {
          n136 = stacked-sequence {
            tunnel: w318 -> [_ w327]
            tunnel: w317 -> [_ w326]
            tunnel: w316 -> [w320 w323]
            tunnel: [_ w325] -> w315
            tunnel: w314 -> [_ w324]
            tunnel: [u32 0 ("Frames in sequence") _] -> w313
            frame #0 {
              n137 = disable-structure shown="Enabled" {
                disable-tunnel: w320 -> [w321 _]
                frame Disabled {
                  n138 = for {
                    tunnel: w321 -> [w322] mode=indexing
                    n139 = Unregister For Events(event registration refnum=w322) -> ()  [unwired: 1 in, 1 out]
                  }
                }
                frame Enabled {
                }
              }
            }
            frame #1 {
              n140 = for {
                tunnel: w327 -> [w332] mode=indexing
                tunnel: w326 -> [w333] mode=indexing
                shift-right: [w331] -> w325
                shift-left: w323 -> [w330]
                tunnel: w324 -> [w329]
                i -> [w328]
                n141 = case shown="True" w333 {
                  tunnel: w332 -> [_ w337]
                  tunnel: [w334 w338] -> w331
                  tunnel: w330 -> [w334 w339]
                  tunnel: w329 -> [_ w336]
                  tunnel: w328 -> [_ w335]
                  frame False {
                  }
                  frame True {
                    n142 = stacked-sequence {
                      tunnel: w339 -> [_ w344 _ _ _ _ _ _ _]
                      tunnel: [_ w345 _ _ _ _ _ _ _] -> w338
                      tunnel: w337 -> [w342 w346 w354 w362 w366 w369 w373 w375 w378]
                      tunnel: w336 -> [_ _ _ w361 _ _ _ _ _]
                      tunnel: w335 -> [_ w343 _ _ _ _ _ _ _]
                      frame #0 {
                        n143 = call <vilib>:"IMAQdx Stop Acquisition.vi"("Session In"=w342) -> ("error out"=w340:errorcluster, "Session Out"=w341:T3)  [unwired: 9 in]
                        n144 = call <vilib>:"IMAQdx Unconfigure Acquisition.vi"("error in"=w340, "Session In"=w341) -> ()  [unwired: 8 in, 2 out]
                      }
                      frame #1 {
                        n145 = disable-structure shown="Enabled" {
                          disable-tunnel: w346 -> [w352 _]
                          disable-tunnel: [w350 w353] -> w345
                          disable-tunnel: w344 -> [w349 w353]
                          disable-tunnel: w343 -> [w347 _]
                          frame Disabled {
                            n146 = register-events(w352, u32 1 ("BufferInterval")) -> (reference out=w348:refnum<event-registration>)  [unwired: 2 in, 1 out]
                            n147 = Replace Array Subset(array=w349, new element=w348, index=w347) -> (w350:refnum<event-registration>[])
                          }
                          frame Enabled {
                          }
                        }
                      }
                      frame #2 {
                        n148 = disable-structure shown="Enabled" {
                          disable-tunnel: w354 -> [w355 w358]
                          frame Disabled {
                            n149 = property class="IMAQdx"(reference=w355, "ActiveAttribute"="CameraAttributes::AcquisitionControl::AcquisitionMode", "ValueU32"=T7."Multi frame") -> ()  [unwired: 1 in, 2 out]
                          }
                          frame Enabled {
                            n150 = property class="IMAQdx"(reference=w358, "ActiveAttribute"="CameraAttributes::AcquisitionControl::AcquisitionMode", "ValueU32"=T7."Continuous") -> ()  [unwired: 1 in, 2 out]
                          }
                        }
                      }
                      frame #3 {
                        n151 = disable-structure shown="Enabled" {
                          disable-tunnel: w362 -> [w364 _]
                          disable-tunnel: w361 -> [w363 _]
                          frame Disabled {
                            n152 = property class="IMAQdx"(reference=w364, "ActiveAttribute"="CameraAttributes::AcquisitionControl::AcquisitionFrameCount", "ValueU32"=w363) -> ()  [unwired: 1 in, 2 out]
                          }
                          frame Enabled {
                          }
                        }
                      }
                      frame #4 {
                        n153 = property class="IMAQdx"(reference=w366, "ActiveAttribute"="CameraAttributes::AcquisitionControl::TriggerSource", "ValueU32"=enum32{"Software", "Line 0", "Line 2", "Line 3"}."Software") -> ()  [unwired: 1 in, 2 out]
                      }
                      frame #5 {
                        n154 = property class="IMAQdx"(reference=w369, "ActiveAttribute"="CameraAttributes::AcquisitionControl::TriggerSelector", "ValueU32"=enum32{"Frame Start", "Exposure Active"}."Frame Start") -> ()  [unwired: 1 in, 2 out]
                      }
                      frame #6 {
                        n155 = property class="IMAQdx"(reference=w373, "ActiveAttribute"="CameraAttributes::AcquisitionControl::TriggerMode", "ValueU32"=enum32{"Off", "On"}."Off") -> ()  [unwired: 1 in, 2 out]
                      }
                      frame #7 {
                        n156 = property class="IMAQdx"(reference=w375, "ActiveAttribute"="CameraAttributes::AcquisitionControl::SingleFrameAcquisitionMode", "ValueU32"=enum16{"Free running", "Triggered"}."Triggered") -> ()  [unwired: 1 in, 2 out]
                      }
                      frame #8 {
                        n157 = disable-structure shown="Enabled" {
                          disable-tunnel: w378 -> [w379 _]
                          frame Disabled {
                            n158 = call <vilib>:"IMAQdx Configure Grab.vi"("Session In"=w379) -> ()  [unwired: 9 in, 2 out]
                          }
                          frame Enabled {
                          }
                        }
                      }
                    }
                  }
                }
              }
            }
          }
        }
      }
      n159 = Bundle By Name(cluster=w234, "Frames to capture"=w236, "Camera event refnums"=w230) -> (w237:T6)
      n160 = To Variant(anything=w237) -> (Variant=w238:variant)
    }
    frame "Set exposure" {
      n161 = Variant To Data(type=w386, Variant=w385) -> (data=w384:T6)  [unwired: 1 in, 1 out]
      n162 = Unbundle By Name(w384) -> ("Camera References"=w381:T3[], "Current camera"=w380:i32)
      n163 = case shown="1, Default" w380 {
        selector: w380 -> [_ w391]
        tunnel: [w389 w394] -> w383
        tunnel: w382 -> [w389 w393]
        tunnel: w381 -> [_ w392]
        frame 65535 {
        }
        frame 1, Default {
          n164 = Decrement(x=w391) -> (x-1=w390:i32)
          n165 = stacked-sequence {
            seq-local: [w399 _] -> [_ w408]
            tunnel: w392 -> [w405 w407]
            tunnel: w393 -> [w397 _]
            tunnel: [_ w409] -> w394
            tunnel: w390 -> [_ _]
            frame #0 {
              n166 = Index Array(array=w405, index=0) -> (element=w406:T3)
              n167 = property class="IMAQdx"(reference=w406, "ActiveAttribute"="CameraAttributes::AcquisitionControl::AutoExposureTimeLowerLimit") -> (reference out=w403:T3, "ValueDBL"=w401:dbl)  [unwired: 1 in, 1 out]
              n168 = Multiply(x=w397, y=1000000.0) -> (x*y=w396:dbl)
              n169 = property class="IMAQdx"(reference=w403, "ActiveAttribute"="CameraAttributes::AcquisitionControl::AutoExposureTimeUpperLimit") -> ("ValueDBL"=w400:dbl)  [unwired: 1 in, 2 out]
              n170 = In Range and Coerce(upper limit=w400, x=w396, lower limit=w401) -> (coerced(x)=w399:dbl)  [unwired: 1 out]
            }
            frame #1 {
              n171 = for {
                tunnel: [w413] -> w409
                tunnel: w408 -> [w411]
                tunnel: w407 -> [w410] mode=indexing
                w412 = "CameraAttributes::AcquisitionControl::ExposureTime"
                n172 = property class="IMAQdx"(reference=w410, "ActiveAttribute"=w412, "ValueDBL"=w411) -> (reference out=w416:T3)  [unwired: 1 in, 1 out]
                n173 = property class="IMAQdx"(reference=w416, "ActiveAttribute"=w412) -> ("ValueDBL"=w414:dbl)  [unwired: 1 in, 2 out]
                n174 = Divide(x=w414, y=1000000.0) -> (x/y=w413:dbl)
              }
            }
          }
        }
      }
      n175 = Bundle By Name(cluster=w388, "Current exposure"=w383) -> (w387:T1)
    }
    frame "Trigger and read" {
      w418 = u32 33 ("Period")
      n176 = Variant To Data(type=w437, Variant=w425) -> (data=w424:T6)  [unwired: 1 in, 1 out]
      n177 = Unbundle By Name(w424) -> ("Camera orientation"=w423:T18, "Current camera"=w432:i32, "Image buffers"=w433:T4[], "Camera References"=w435:T3[], "Camera event refnums"=w434:refnum<event-registration>[], "Frames to capture"=w436:u32, "File write access"=w426:T5, "RGB Channels"=w420:T19, "RGB buffers"=w419:T4[])
      n178 = Variant To Data(type=T9 {"New Image"=refnum, "Image"=refnum, "FPS target"=30.0} ("output cluster"), Variant=w429) -> (data=w431:T9)  [unwired: 1 in, 1 out]
      n179 = Unbundle(w431) -> ("New Image"=w428:T4, "Image"=w427:refnum<vi>)  [unwired: 1 out]
      n180 = To Quad Integer(1:w418) -> (0:w417:i64)
      n181 = case shown="2, Default" w436 {
        selector: w436 -> [_ w637]
        tunnel: w438 -> [w444 w643]
        tunnel: w428 -> [w445 w642]
        tunnel: w435 -> [w448 w641]
        tunnel: w434 -> [_ w640]
        tunnel: w433 -> [w447 w639]
        tunnel: w432 -> [w446 w638]
        tunnel: w427 -> [w443 w636]
        tunnel: w426 -> [_ w635]
        tunnel: w424 -> [w441 w634]
        tunnel: w423 -> [w442 w633]
        tunnel: [w440 w632] -> w422
        tunnel: w421 -> [_ w631]
        tunnel: w420 -> [_ w630]
        tunnel: w419 -> [_ w629]
        tunnel: w418 -> [_ w628]
        tunnel: w417 -> [_ w627]
        tunnel: w418 -> [_ w626]
        frame 0 {
          n182 = stacked-sequence {
            tunnel: w448 -> [w455 _]
            tunnel: w447 -> [w453 w547]
            tunnel: w446 -> [w452 _]
            tunnel: w445 -> [w451 w544]
            tunnel: w444 -> [w450 _]
            tunnel: w441 -> [_ w546]
            tunnel: w443 -> [_ w545]
            tunnel: w442 -> [w449 _]
            frame #0 {
              n183 = Array Size(array=w453) -> (size(s)=w454:i32)
              n184 = for {
                tunnel: w453 -> [w468] mode=indexing
                tunnel: w455 -> [w469] mode=indexing
                workers-P: w454 -> [_]
                tunnel: w452 -> [w467]
                tunnel: w451 -> [w464]
                tunnel: w450 -> [w460]
                tunnel: w449 -> [w456] mode=indexing
                i -> [w466]
                n185 = Decrement(x=w467) -> (x-1=w459:i32)
                n186 = Equal?(x=w459, y=w466) -> (x = y?=w465:bool)
                n187 = call <vilib>:"IMAQdx Snap2.vi"("Image In"=w468, "Session In"=w469) -> ("Image Out"=w458:T4)  [unwired: 7 in, 2 out]
                n188 = case shown="\"Clockwise, Flip LR\"" w456 {
                  tunnel: w458 -> [w470 w473 w476 w479 w486 w493 w496 w505 w512]
                  tunnel: [w470 w472 w475 w477 w482 w489 w497 w501 w508] -> w457
                  frame "No rotation, No flip", Default {
                  }
                  frame "No rotation, Flip UD" {
                    w471 = u32 0 items=["Horizontal", "Vertical", "Central", "1st Diagonal", "2nd Diagonal"] ("Type of Symmetry")
                    n189 = call "IMAQ Symmetry"("Type of Symmetry"=w471, "Image Dst"=w473, "Image Src"=w473) -> ("Image Dst Out"=w472:T4)  [unwired: 2 in, 1 out]
                  }
                  frame "No rotation, Flip LR" {
                    w474 = u32 1 items=["Horizontal", "Vertical", "Central", "1st Diagonal", "2nd Diagonal"] ("Type of Symmetry")
                    n190 = call "IMAQ Symmetry"("Type of Symmetry"=w474, "Image Dst"=w476, "Image Src"=w476) -> ("Image Dst Out"=w475:T4)  [unwired: 2 in, 1 out]
                  }
                  frame "Clockwise, No flip" {
                    n191 = call "IMAQ Rotate"("Use Bilinear Interpolation"=FALSE, "Maintain Size"=FALSE, "Angle (degrees)"=sgl 270.0, "Image Dst"=w479, "Image Src"=w479) -> ("Image Dst Out"=w477:T4)  [unwired: 5 in, 1 out]
                  }
                  frame "Clockwise, Flip UD" {
                    w484 = u32 0 items=["Horizontal", "Vertical", "Central", "1st Diagonal", "2nd Diagonal"] ("Type of Symmetry")
                    n192 = call "IMAQ Rotate"("Use Bilinear Interpolation"=FALSE, "Maintain Size"=FALSE, "Angle (degrees)"=sgl 270.0, "Image Dst"=w486, "Image Src"=w486) -> ("Image Dst Out"=w483:T4)  [unwired: 5 in, 1 out]
                    n193 = call "IMAQ Symmetry"("Type of Symmetry"=w484, "Image Dst"=w483, "Image Src"=w483) -> ("Image Dst Out"=w482:T4)  [unwired: 2 in, 1 out]
                  }
                  frame "Clockwise, Flip LR" {
                    w491 = u32 1 items=["Horizontal", "Vertical", "Central", "1st Diagonal", "2nd Diagonal"] ("Type of Symmetry")
                    n194 = call "IMAQ Rotate"("Use Bilinear Interpolation"=FALSE, "Maintain Size"=FALSE, "Angle (degrees)"=sgl 270.0, "Image Dst"=w493, "Image Src"=w493) -> ("Image Dst Out"=w490:T4)  [unwired: 5 in, 1 out]
                    n195 = call "IMAQ Symmetry"("Type of Symmetry"=w491, "Image Dst"=w490, "Image Src"=w490) -> ("Image Dst Out"=w489:T4)  [unwired: 2 in, 1 out]
                  }
                  frame "Anticlockwise, No flip" {
                    n196 = call "IMAQ Rotate"("Use Bilinear Interpolation"=FALSE, "Maintain Size"=FALSE, "Angle (degrees)"=sgl 90.0, "Image Dst"=w496, "Image Src"=w496) -> ("Image Dst Out"=w497:T4)  [unwired: 5 in, 1 out]
                  }
                  frame "Anticlockwise, Flip UD" {
                    w503 = u32 0 items=["Horizontal", "Vertical", "Central", "1st Diagonal", "2nd Diagonal"] ("Type of Symmetry")
                    n197 = call "IMAQ Rotate"("Use Bilinear Interpolation"=FALSE, "Maintain Size"=FALSE, "Angle (degrees)"=sgl 90.0, "Image Dst"=w505, "Image Src"=w505) -> ("Image Dst Out"=w502:T4)  [unwired: 5 in, 1 out]
                    n198 = call "IMAQ Symmetry"("Type of Symmetry"=w503, "Image Dst"=w502, "Image Src"=w502) -> ("Image Dst Out"=w501:T4)  [unwired: 2 in, 1 out]
                  }
                  frame "Anticlockwise, Flip LR" {
                    w510 = u32 1 items=["Horizontal", "Vertical", "Central", "1st Diagonal", "2nd Diagonal"] ("Type of Symmetry")
                    n199 = call "IMAQ Rotate"("Use Bilinear Interpolation"=FALSE, "Maintain Size"=FALSE, "Angle (degrees)"=sgl 90.0, "Image Dst"=w512, "Image Src"=w512) -> ("Image Dst Out"=w509:T4)  [unwired: 5 in, 1 out]
                    n200 = call "IMAQ Symmetry"("Type of Symmetry"=w510, "Image Dst"=w509, "Image Src"=w509) -> ("Image Dst Out"=w508:T4)  [unwired: 2 in, 1 out]
                  }
                }
                n201 = case shown="True" w465 {
                  tunnel: w457 -> [_ w542]
                  tunnel: w464 -> [_ w543]
                  frame False {
                  }
                  frame True {
                    n202 = call "IMAQ Copy"("Image Dst"=w543, "Image Src"=w542) -> ()  [unwired: 4 in, 2 out]
                  }
                }
                n203 = call "IMAQ GetImageSize"("Image"=w457) -> ("Y Resolution"=w461:i32, "X Resolution"=w462:i32)  [unwired: 3 in, 1 out]
                n204 = Not A Number/Path/Refnum?(number/path/refnum=w460) -> (NaN/Path/Refnum?=w463:bool)
                n205 = case shown="False" w463 {
                  tunnel: w460 -> [w518 _]
                  tunnel: w457 -> [w519 _]
                  tunnel: w462 -> [w516 _]
                  tunnel: w461 -> [w515 _]
                  frame False {
                    n206 = call <vilib>:"Get File Extension.vi"("file"=w518) -> ("lowercase file extension"=w517:string)  [unwired: 6 in, 4 out]
                    n207 = case shown="\"dat\", \"u16\"" w517 {
                      tunnel: w518 -> [w532 w541 _]
                      tunnel: w519 -> [w522 w536 _]
                      tunnel: w516 -> [w530 _ _]
                      tunnel: w515 -> [w529 _ _]
                      frame "'tiff'", "tif" {
                        n208 = call "TIFFStream Open.vi"("Bytes per strip"=u32 8000, "File path"=w532, "Height Pixels"=w529, "Width Pixels"=w530, "Big endian?"=FALSE) -> ("error out"=w526:errorcluster, "Current and next IFD offset"=w524:u32[], "Image data reference"=w523:refnum<data-value>, "File data"=w528:T11)  [unwired: 3 in]
                        n209 = in-place {
                          in-place-border: w522 -> [w534]
                          n210 = in-place-dvr #1(w523) -> ()  [unwired: 2 out]
                          n211 = call "IMAQ ImageToArray"("Image"=w534) -> ("Image Pixels (I16)"=w533:i16[][])  [unwired: 3 in, 4 out]
                          n212 = in-place-dvr #1(w533) -> (w520:refnum<data-value>)  [unwired: 1 out]
                        }
                        n213 = call "TIFFStream Write.vi"("File data"=w528, "error in (no error)"=w526, "Last image in file?"=TRUE, "Current and next IFD offset in"=w524, "Image data reference"=w520) -> ("error out"=w527:errorcluster)  [unwired: 4 in, 2 out]
                        n214 = call "TIFFStream Close.vi"("error in (no error)"=w527, "Image data reference"=w520, "File data"=w528) -> ()  [unwired: 8 in, 1 out]
                      }
                      frame "dat", "u16" {
                        # "No need to cast - no negative values"
                        n215 = Open/Create/Replace File(file path (use dialog)=w541, operation (0:open)=T10."replace or create") -> (refnum out=w540:refnum<file>)  [unwired: 4 in, 2 out]
                        n216 = call "IMAQ ImageToArray"("Image"=w536) -> ("Image Pixels (I16)"=w535:i16[][])  [unwired: 3 in, 4 out]
                        n217 = Write to Binary File(file (use dialog)=w540, data=w535, 5:FALSE ("prepend array or string size? (T)")) -> (refnum out=w538:refnum<file>)  [unwired: 3 in, 2 out]
                        n218 = Close File(refnum=w538) -> ()  [unwired: 1 in, 2 out]
                      }
                      frame "None", Default {
                      }
                    }
                  }
                  frame True {
                  }
                }
              }
            }
            frame #1 {
              n219 = Unbundle By Name(w546) -> ("Offset and gain"=w551:dbl[][], "RGB Channels"=w550:T19, "RGB buffers"=w549:T4[], "Current camera"=w548:i32)
              n220 = case shown="0" w548 {
                tunnel: w551 -> [_ w576]
                tunnel: w550 -> [_ w575]
                tunnel: w547 -> [_ w574]
                tunnel: w549 -> [_ w572]
                tunnel: w545 -> [_ w570]
                tunnel: w544 -> [_ w556]
                frame 1, Default {
                }
                frame 0 {
                  w555 = 0 ("X Resolution")
                  w561 = u16 0 items=["RGB", "HSL", "HSV", "HSI"] ("Color Mode")
                  n221 = Index Array(array=w572, index #1=0 ("index"), index #2=1 ("index")) -> (element #1=w552:T4, element #2=w568:T4)
                  n222 = Array Subset(array=w572, index=2 ("length"), length=3 ("index")) -> (w573:T4[])
                  n223 = for {
                    tunnel: w573 -> [w587] mode=indexing
                    tunnel: w576 -> [w586] mode=indexing
                    tunnel: w575 -> [w589] mode=indexing
                    tunnel: w574 -> [w588]
                    tunnel: [w585] -> w567 mode=indexing
                    tunnel: w568 -> [w584]
                    shift-right: [w580] -> w554
                    shift-left: w555 -> [w583]
                    shift-right: [w581] -> w553
                    shift-left: w555 -> [w582]
                    tunnel: w552 -> [w579]
                    n224 = case shown="\"None\"" w589 {
                      selector: w589 -> [_ w625]
                      tunnel: w588 -> [_ w624]
                      tunnel: w587 -> [w593 w610]
                      tunnel: w586 -> [_ w620]
                      tunnel: [w599 w609] -> w585
                      tunnel: w584 -> [_ w622]
                      tunnel: w583 -> [w597 w605]
                      tunnel: w582 -> [w595 w603]
                      tunnel: [w595 w602] -> w581
                      tunnel: [w597 w601] -> w580
                      tunnel: w579 -> [w598 _]
                      frame "None" {
                        n225 = call "IMAQ GetImageSize"("Image"=w598) -> ("Y Resolution"=w594:i32, "X Resolution"=w596:i32)  [unwired: 3 in, 1 out]
                        n226 = Max & Min(x=w597, y=w596) -> (max(x,y)=w591:i32)  [unwired: 1 out]
                        n227 = Max & Min(x=w595, y=w594) -> (max(x,y)=w590:i32)  [unwired: 1 out]
                        n228 = call "IMAQ SetImageSize"("Y Resolution"=w590, "X Resolution"=w591, "Image"=w593) -> ("Image Out"=w592:T4)  [unwired: 2 in, 1 out]
                        n229 = call "IMAQ FillImage"("Pixel Value (U8, U16, I16, Float)"=sgl 0.0, "Image"=w592) -> ("Image Out"=w599:T4)  [unwired: 8 in, 1 out]
                      }
                      frame "Camera 1", Default {
                        w611 = T17 0 items=["Grayscale (U8)", "Grayscale (I16)", "Grayscale (SGL)", "Complex (CSG)", "RGB (U32)", "HSL (U32)", "RGB (U64)", "Grayscale (U16)"] ("Image Type")
                        w621 = T17 2 items=["Grayscale (U8)", "Grayscale (I16)", "Grayscale (SGL)", "Complex (CSG)", "RGB (U32)", "HSL (U32)", "RGB (U64)", "Grayscale (U16)"] ("Image Type")
                        n230 = Decrement(x=w625) -> (x-1=w623:T21)
                        n231 = Index Array(array=w624, index=w623) -> (element=w608:T4)
                        n232 = call "IMAQ GetImageSize"("Image"=w608) -> ("Y Resolution"=w604:i32, "X Resolution"=w606:i32, "error out"=w607:errorcluster)  [unwired: 3 in]
                        n233 = Index Array(array=w620, index #1=0 ("index"), index #2=1 ("index")) -> (element #1=w617:dbl, element #2=w613:dbl)
                        n234 = call "IMAQ Cast Image"("Image Type"=w621, "error in (no error)"=w607, "Image Dst"=w622, "Image Src"=w608) -> ("Image Dst Out"=w616:T4)  [unwired: 6 in, 1 out]
                        n235 = Max & Min(x=w605, y=w606) -> (max(x,y)=w601:i32)  [unwired: 1 out]
                        n236 = Max & Min(x=w603, y=w604) -> (max(x,y)=w602:i32)  [unwired: 1 out]
                        n237 = call "IMAQ Add"("Image Src A"=w616, "Constant"=w617, "Image Dst"=w616) -> ("Image Dst Out"=w614:T4, "error out"=w615:errorcluster)  [unwired: 4 in]
                        n238 = call "IMAQ Multiply"("Image Src A"=w614, "Constant"=w613, "Image Dst"=w614, "error in (no error)"=w615) -> ("Image Dst Out"=w612:T4)  [unwired: 3 in, 1 out]
                        n239 = call "IMAQ Cast Image"("Image Type"=w611, "Image Dst"=w610, "Image Src"=w612) -> ("Image Dst Out"=w609:T4)  [unwired: 7 in, 1 out]
                      }
                    }
                  }
                  n240 = Index Array(array=w567, index #1=0 ("index"), index #2=1 ("index"), index #3=2 ("index")) -> (element #1=w559:T4, element #2=w563:T4, element #3=w562:T4)
                  n241 = call "IMAQ SetImageSize"("Y Resolution"=w553, "X Resolution"=w554, "Image"=w552) -> ("Image Out"=w560:T4)  [unwired: 2 in, 1 out]
                  n242 = call "IMAQ ReplaceColorPlane"("Image Src"=w560, "Color Mode"=w561, "Image Dst"=w560, "Red or Hue Plane"=w559, "Green or Sat Plane"=w563, "Blue or Luma or Val or Inten Plane"=w562) -> ("Image Dst Out"=w558:T4)  [unwired: 8 in, 1 out]
                  n243 = call "IMAQ Copy"("Image Dst"=w556, "Image Src"=w558) -> ("Image Dst Out"=w557:T4)  [unwired: 4 in, 1 out]
                  n244 = property class="ImageControl"(reference=w570, "Value"=w557) -> ()  [unwired: 1 in, 2 out]
                }
              }
            }
          }
          n245 = To Variant(anything=w441) -> (Variant=w440:variant)
        }
        frame 2, Default {
          n246 = stacked-sequence {
            seq-local: [w665 _ _ _] -> [_ _ w766 w1704]
            seq-local: [w664 _ _ _] -> [_ _ w765 w1703]
            seq-local: [w644 _ _ _] -> [_ _ w764 w1702]
            seq-local: [w663 _ _ _] -> [_ _ w763 w1701]
            seq-local: [w662 _ _ _] -> [_ _ w762 w1698]
            seq-local: [w655 _ _ _] -> [_ _ w745 w1700]
            seq-local: [w649 _ _ _] -> [_ _ w739 _]
            tunnel: w643 -> [w667 _ w761 w1699]
            tunnel: w642 -> [_ _ w746 _]
            tunnel: w641 -> [w650 w724 w768 w1705]
            tunnel: w640 -> [w651 _ _ _]
            tunnel: w639 -> [_ _ w750 _]
            tunnel: w638 -> [_ _ w760 _]
            tunnel: w637 -> [_ _ w742 _]
            tunnel: w636 -> [_ _ w747 _]
            tunnel: w635 -> [_ _ w759 _]
            tunnel: w634 -> [w654 _ w749 _]
            tunnel: w633 -> [_ _ w744 _]
            tunnel: [w653 _ _ _] -> w632
            tunnel: w631 -> [_ _ w738 _]
            tunnel: w630 -> [_ _ w737 _]
            tunnel: w629 -> [_ _ w736 _]
            tunnel: w628 -> [_ _ w735 _]
            tunnel: w627 -> [_ _ w734 _]
            tunnel: w626 -> [_ _ w733 _]
            frame #0 {
              # "Start acquisition"
              n247 = Index Array(array=w650, index=0) -> (element=w658:T3)
              n248 = for {
                tunnel: w651 -> [w671] mode=indexing
                tunnel: [w669] -> w649 mode=indexing
                tunnel: w650 -> [w670] mode=indexing
                n249 = Unregister For Events(event registration refnum=w671) -> ()  [unwired: 1 in, 1 out]
                n250 = register-events(w670, u32 1 ("BufferInterval")) -> (reference out=w669:refnum<event-registration>)  [unwired: 2 in, 1 out]
              }
              n251 = property class="IMAQdx"(reference=w658, "ActiveAttribute"="CameraAttributes::ImageFormatControl::Width") -> ("ValueU32"=w660:u32)  [unwired: 1 in, 2 out]
              n252 = property class="IMAQdx"(reference=w658, "ActiveAttribute"="CameraAttributes::ImageFormatControl::Height") -> ("ValueU32"=w656:u32)  [unwired: 1 in, 2 out]
              n253 = Not A Number/Path/Refnum?(number/path/refnum=w667) -> (NaN/Path/Refnum?=w666:bool)
              n254 = case shown="False" w666 {
                tunnel: w667 -> [w680 _]
                tunnel: w660 -> [w679 _]
                tunnel: w656 -> [w678 _]
                tunnel: [w677 T11 {"File refnum"=refnum, "Image File Directory"={[], []}, "Big endian?"=FALSE, "IFD Offset Size"=0} ("File data")] -> w645
                tunnel: [w676 refnum<data-value> refnum ("Image data reference")] -> w663
                tunnel: [w675 refnum<queue> refnum ("queue out")] -> w662
                tunnel: [w674 refnum<file> refnum ("refnum out")] -> w664
                tunnel: [w673 "None" ("lowercase file extension")] -> w665
                tunnel: [w672 refnum<queue> refnum ("queue out")] -> w655
                frame False {
                  n255 = call <vilib>:"Get File Extension.vi"("file"=w680) -> ("lowercase file extension"=w673:string)  [unwired: 6 in, 4 out]
                  n256 = case shown="\"'tiff'\", \"tif\"" w673 {
                    tunnel: w680 -> [w700 w712 _]
                    tunnel: w679 -> [w698 _ _]
                    tunnel: w678 -> [w697 _ _]
                    tunnel: [w695 T11 {"File refnum"=refnum, "Image File Directory"={[], []}, "Big endian?"=FALSE, "IFD Offset Size"=0} ("File data") T11 {"File refnum"=refnum, "Image File Directory"={[], []}, "Big endian?"=FALSE, "IFD Offset Size"=0} ("File data")] -> w677
                    tunnel: [w694 refnum<data-value> refnum ("Image data reference") refnum<data-value> refnum ("Image data reference")] -> w676
                    tunnel: [w687 refnum<queue> refnum ("queue out") refnum<queue> refnum ("queue out")] -> w675
                    tunnel: [refnum<file> refnum ("refnum out") w710 refnum<file> refnum ("refnum out")] -> w674
                    tunnel: [w684 w701 refnum<queue> refnum ("queue out")] -> w672
                    frame "'tiff'", "tif" {
                      # "Hack to deal with poor stripe handling"
                      n257 = call "TIFFStream Open.vi"("Bytes per strip"=u32 128000000, "File path"=w700, "Height Pixels"=w697, "Width Pixels"=w698, "Big endian?"=FALSE) -> ("Current and next IFD offset"=w689:u32[], "Image data reference"=w694:refnum<data-value>, "File data"=w695:T11)  [unwired: 3 in, 1 out]
                      n258 = Obtain Queue(max queue size (-1, unlimited)=1, name (unnamed)="TIFF position", element data type=w689) -> (queue out=w688:refnum<queue>, error out=w690:errorcluster)  [unwired: 2 in, 1 out]
                      n259 = Lossy Enqueue Element(queue=w688, element=w689, error in (no error)=w690) -> (queue out=w687:refnum<queue>)  [unwired: 3 out]
                      n260 = Bundle("Camera identity"=enum16{"Camera 1", "Camera 2", "Camera 3"}."Camera 1", "Timestamp"=u64 0) -> (w681:T22)  [unwired: 1 in]
                      n261 = Obtain Queue(max queue size (-1, unlimited)=-1, name (unnamed)="PG Frame order", element data type=w681) -> (queue out=w684:refnum<queue>)  [unwired: 2 in, 2 out]
                    }
                    frame "dat", "u16" {
                      n262 = Bundle("Camera identity"=enum16{"Camera 1", "Camera 2", "Camera 3"}."Camera 1", "Timestamp"=u64 0) -> (w702:T22)  [unwired: 1 in]
                      n263 = Open/Create/Replace File(file path (use dialog)=w712, operation (0:open)=T10."replace or create") -> (refnum out=w710:refnum<file>)  [unwired: 4 in, 2 out]
                      n264 = Obtain Queue(max queue size (-1, unlimited)=-1, name (unnamed)="PG Frame order", element data type=w702) -> (queue out=w701:refnum<queue>)  [unwired: 2 in, 2 out]
                    }
                    frame "None", Default {
                    }
                  }
                }
                frame True {
                }
              }
              n265 = Bundle By Name(cluster=w654, "Camera event refnums"=w649) -> (w652:T6)
              n266 = To Variant(anything=w652) -> (Variant=w653:variant)
              n267 = Obtain Queue(max queue size (-1, unlimited)=1, name (unnamed)="PG TIFF File Data", element data type=w645) -> (queue out=w646:refnum<queue>)  [unwired: 2 in, 2 out]
              n268 = Lossy Enqueue Element(queue=w646, element=w645) -> (queue out=w644:refnum<queue>)  [unwired: 1 in, 3 out]
            }
            frame #1 {
              n269 = for {
                tunnel: w724 -> [w725] mode=indexing
                n270 = disable-structure shown="Enabled" {
                  disable-tunnel: w725 -> [w727 w732]
                  frame Disabled {
                    n271 = property class="IMAQdx"(reference=w727, "ActiveAttribute"="CameraAttributes::AcquisitionControl::TriggerSoftware") -> ()  [unwired: 1 in, 2 out]
                  }
                  frame Enabled {
                    n272 = call <vilib>:"IMAQdx Configure Acquisition.vi"("Number of Buffers"=u32 5, "Continuous?"=IMAQdx_Acquisition_Mode."Continuous", "Session In"=w732) -> ("error out"=w728:errorcluster, "Session Out"=w731:T3)  [unwired: 7 in]
                    n273 = call <vilib>:"IMAQdx Start Acquisition.vi"("error in"=w728, "Session In"=w731) -> ()  [unwired: 8 in, 2 out]
                  }
                }
              }
            }
            frame #2 {
              n274 = Obtain Notifier(name (unnamed)="PG Colour", notification data type=FALSE) -> (notifier out=w756:refnum<notifier>, error out=w751:errorcluster)  [unwired: 2 in, 1 out]
              n275 = In Range and Coerce(upper limit=u32 4294967295, x=w742, lower limit=u32 0) -> (coerced(x)=w743:u32)  [unwired: 1 out]
              n276 = Send Notification(notification=FALSE, notifier=w756, error in (no error)=w751) -> (notifier out=w753:refnum<notifier>)  [unwired: 1 out]
              n277 = To Long Integer(number=w743) -> (32bit integer=w767:i32)
              n278 = stacked-sequence {
                tunnel: w739 -> [w909 _]
                tunnel: w768 -> [w897 _]
                tunnel: w750 -> [w896 _]
                tunnel: w767 -> [w873 _]
                tunnel: w766 -> [w874 _]
                tunnel: w765 -> [w875 _]
                tunnel: w764 -> [w876 _]
                tunnel: w763 -> [w877 _]
                tunnel: w762 -> [w871 _]
                tunnel: w761 -> [w868 _]
                tunnel: w760 -> [w864 _]
                tunnel: w746 -> [w863 _]
                tunnel: w747 -> [w862 _]
                tunnel: w759 -> [w861 _]
                tunnel: w753 -> [_ w1697]
                tunnel: w745 -> [w878 _]
                tunnel: w744 -> [w890 _]
                tunnel: w738 -> [w859 _]
                tunnel: w737 -> [w865 _]
                tunnel: w736 -> [w888 _]
                tunnel: w735 -> [w885 _]
                tunnel: w733 -> [w867 _]
                frame #0 {
                  n279 = Array Subset(array=w888, index=5, length=3 ("index")) -> (w860:T4[])
                  n280 = Index Array(array=w909, index #1=0 ("index"), index #2=1 ("index"), index #3=2 ("index")) -> (element #1=w894:refnum<event-registration>, element #2=w880:refnum<event-registration>, element #3=w866:refnum<event-registration>)
                  n281 = Index Array(array=w890, index #1=0 ("index"), index #2=1 ("index"), index #3=2 ("index")) -> (element #1=w889:T23, element #2=w883:T23, element #3=w872:T23)
                  n282 = Index Array(array=w896, index #1=0 ("index"), index #2=1 ("index"), index #3=2 ("index")) -> (element #1=w902:T4, element #2=w882:T4, element #3=w870:T4)
                  n283 = Index Array(array=w897, index #1=0 ("index"), index #2=1 ("index"), index #3=2 ("index")) -> (element #1=w898:T3, element #2=w881:T3, element #3=w869:T3)
                  n284 = Not A Number/Path/Refnum?(number/path/refnum=w894) -> (NaN/Path/Refnum?=w895:bool)
                  n285 = Not A Number/Path/Refnum?(number/path/refnum=w880) -> (NaN/Path/Refnum?=w884:bool)
                  n286 = Not A Number/Path/Refnum?(number/path/refnum=w866) -> (NaN/Path/Refnum?=w879:bool)
                  n287 = case shown="False" w884 {
                    tunnel: w880 -> [w1192 _]
                    tunnel: w882 -> [w1191 _]
                    tunnel: w881 -> [w1190 _]
                    tunnel: w873 -> [w1189 _]
                    tunnel: w874 -> [w1188 _]
                    tunnel: w875 -> [w1187 _]
                    tunnel: w876 -> [w1186 _]
                    tunnel: w877 -> [w1185 _]
                    tunnel: w871 -> [w1184 _]
                    tunnel: w868 -> [w1183 _]
                    tunnel: w864 -> [w1182 _]
                    tunnel: w863 -> [w1181 _]
                    tunnel: w862 -> [w1180 _]
                    tunnel: w861 -> [w1179 _]
                    tunnel: w878 -> [w1178 _]
                    tunnel: w883 -> [w1177 _]
                    tunnel: w859 -> [w1176 _]
                    tunnel: w865 -> [w1175 _]
                    tunnel: w860 -> [w1174 _]
                    tunnel: w867 -> [w1172 _]
                    frame False {
                      n288 = for {
                        N: w1189 -> [_]
                        tunnel: w1183 -> [w1213]
                        tunnel: w1181 -> [w1212]
                        tunnel: w1192 -> [w1211]
                        tunnel: w1190 -> [w1210]
                        tunnel: w1191 -> [w1209]
                        tunnel: w1182 -> [w1208]
                        tunnel: w1187 -> [w1206]
                        tunnel: w1188 -> [w1205]
                        tunnel: w1186 -> [w1204]
                        tunnel: w1185 -> [w1203]
                        tunnel: w1180 -> [w1202]
                        tunnel: w1184 -> [w1201]
                        tunnel: w1179 -> [w1200]
                        tunnel: w1178 -> [w1199]
                        tunnel: w1177 -> [w1198]
                        tunnel: w1176 -> [w1197]
                        border: u32 0 ("millisecond timer value") -> [_]
                        tunnel: w1175 -> [w1195]
                        tunnel: w1174 -> [w1194]
                        tunnel: w1172 -> [w1193]
                        stop <- w1196 stop-if-true
                        n289 = event shown="[1] <Session Out>: Frame Done" {
                          selector: w1211 -> [_ _]
                          dyn-events: _ -> [_ _]
                          timeout: 1000 -> [_ _]
                          tunnel: w1213 -> [_ _]
                          tunnel: w1212 -> [_ w1247]
                          tunnel: w1210 -> [_ w1241]
                          tunnel: w1209 -> [_ w1237]
                          tunnel: w1208 -> [_ w1240]
                          tunnel: w1206 -> [_ w1245]
                          tunnel: w1205 -> [_ w1217]
                          tunnel: w1204 -> [_ w1244]
                          tunnel: w1203 -> [_ w1243]
                          tunnel: w1202 -> [_ w1242]
                          tunnel: w1201 -> [_ w1238]
                          tunnel: w1200 -> [_ w1234]
                          tunnel: w1199 -> [_ w1239]
                          tunnel: w1198 -> [_ w1222]
                          tunnel: w1197 -> [w1216 w1233]
                          tunnel: [w1214 w1235] -> w1196
                          tunnel: w1195 -> [_ w1220]
                          tunnel: w1194 -> [_ w1219]
                          tunnel: w1193 -> [_ w1218]
                          event Timeout {
                            n290 = event-data() -> ()  [unwired: 1 in, 3 out]
                            n291 = property class="Bool (strict)"(reference=w1216) -> ("Value"=w1215:bool)  [unwired: 1 in, 2 out]
                            n292 = Not(x=w1215) -> (.not. x?=w1214:bool)
                          }
                          event event #0x0 {
                            # "Read data"
                            n293 = event-data() -> ()  [unwired: 1 in, 1 out]
                            n294 = Tick Count (ms)() -> (millisecond timer value=w1221:u32)
                            n295 = feedback #2() -> (w1230:u32)
                            n296 = call "Elapsed time.vi"("Start time (ms)"=w1230, "Current time (ms)"=w1221) -> ("Elapsed time"=w1232:u32)
                            n297 = Greater?(x=w1232, y=w1218) -> (0:w1226:bool)
                            n298 = Select(t=w1221, s=w1226, f=w1230) -> (s? t:f=w1231:u32)
                            n299 = feedback-in #2(w1231) -> ()
                            n300 = call <vilib>:"IMAQdx Get Image2.vi"("Buffer Number Mode (Next)"=IMAQdx_Buffer_Number_Mode."Last New", "Image In"=w1237, "Session In"=w1241) -> ("error out"=w1224:errorcluster, "Image Out"=w1225:T4)  [unwired: 5 in, 2 out]
                            n301 = Not A Number/Path/Refnum?(number/path/refnum=w1247) -> (NaN/Path/Refnum?=w1228:bool)
                            n302 = Not(x=w1226) -> (.not. x?=w1227:bool)
                            n303 = Or(x=w1228, y=w1227) -> (x .or. y?=w1229:bool)
                            n304 = case shown="\"dat\", \"u16\"" w1217 {
                              tunnel: w1225 -> [w1249 w1293 w1296]
                              tunnel: w1245 -> [_ _ w1297]
                              tunnel: w1244 -> [w1250 _ _]
                              tunnel: w1243 -> [w1251 _ _]
                              tunnel: w1238 -> [w1255 _ _]
                              tunnel: w1234 -> [w1254 _ w1301]
                              tunnel: w1239 -> [w1253 _ w1298]
                              tunnel: w1224 -> [w1252 _ w1300]
                              tunnel: [w1248 w1293 w1296] -> w1223
                              frame "'tiff'", "tif" {
                                n305 = stacked-sequence {
                                tunnel: w1255 -> [_ w1269 _ _]
                                tunnel: w1254 -> [w1256 _ _ w1286]
                                tunnel: w1253 -> [_ _ w1284 _]
                                tunnel: w1252 -> [_ w1264 _ _]
                                tunnel: w1251 -> [_ w1263 _ _]
                                tunnel: w1250 -> [_ w1259 _ _]
                                tunnel: w1249 -> [_ w1261 w1275 _]
                                tunnel: [_ w1261 _ _] -> w1248
                                frame #0 {
                                n306 = call <vilib>:"Acquire Semaphore.vi"("semaphore"=w1256) -> ()  [unwired: 4 in, 3 out]
                                }
                                frame #1 {
                                n307 = Preview Queue Element(queue=w1259) -> (queue out=w1260:refnum<queue>, element=w1258:T11)  [unwired: 2 in, 2 out]
                                n308 = in-place {
                                in-place-border: w1261 -> [w1272]
                                in-place-border: w1264 -> [w1271]
                                n309 = in-place-dvr #3(w1263) -> ()  [unwired: 2 out]
                                n310 = call "IMAQ ImageToArray"("error in (no error)"=w1271, "Image"=w1272) -> ("Image Pixels (I16)"=w1270:i16[][])  [unwired: 2 in, 4 out]
                                n311 = in-place-dvr #3(w1270) -> (w1262:refnum<data-value>)  [unwired: 1 out]
                                }
                                n312 = Preview Queue Element(queue=w1269) -> (queue out=w1267:refnum<queue>, element=w1268:u32[])  [unwired: 2 in, 2 out]
                                n313 = call "TIFFStream Write.vi"("File data"=w1258, "Last image in file?"=FALSE, "Current and next IFD offset in"=w1268, "Image data reference"=w1262) -> ("Current and next IFD offset out"=w1266:u32[], "File data out"=w1257:T11)  [unwired: 5 in, 1 out]
                                n314 = Lossy Enqueue Element(queue=w1260, element=w1257) -> ()  [unwired: 1 in, 4 out]
                                n315 = Lossy Enqueue Element(queue=w1267, element=w1266) -> ()  [unwired: 1 in, 4 out]
                                }
                                frame #2 {
                                w1278 = u32 0
                                n316 = call "IMAQ Read Custom Data"("Key"="IMAQdxReceiveTimestampHigh", "Image"=w1275) -> ("Custom Data Out"=w1282:string, "Image (duplicate)"=w1281:T4)  [unwired: 7 in, 1 out]
                                n317 = Unflatten From String(type=w1278, binary string=w1282) -> (value=w1277:u32)  [unwired: 3 in, 2 out]
                                n318 = call "IMAQ Read Custom Data"("Key"="IMAQdxReceiveTimestampLow", "Image"=w1281) -> ("Custom Data Out"=w1279:string)  [unwired: 7 in, 2 out]
                                n319 = Unflatten From String(type=w1278, binary string=w1279) -> (value=w1276:u32)  [unwired: 3 in, 2 out]
                                n320 = Join Numbers(hi=w1277, lo=w1276) -> ((hi.lo)=w1273:u64)
                                n321 = Bundle("element"=enum16{"Camera 1", "Camera 2", "Camera 3"}."Camera 2", w1273) -> (w1274:T24)  [unwired: 1 in]
                                n322 = Enqueue Element(queue=w1284, element=w1274) -> ()  [unwired: 2 in, 3 out]
                                }
                                frame #3 {
                                n323 = call <vilib>:"Release Semaphore.vi"("semaphore"=w1286) -> ()  [unwired: 5 in, 2 out]
                                }
                                }
                              }
                              frame "None", Default {
                                w1289 = u32 0
                                n324 = call "IMAQ Read Custom Data"("Key"="IMAQdxReceiveTimestampHigh", "Image"=w1293) -> ("Custom Data Out"=w1294:string, "Image (duplicate)"=w1292:T4)  [unwired: 7 in, 1 out]
                                n325 = Unflatten From String(type=w1289, binary string=w1294) -> (value=w1288:u32)  [unwired: 3 in, 2 out]
                                n326 = call "IMAQ Read Custom Data"("Key"="IMAQdxReceiveTimestampLow", "Image"=w1292) -> ("Custom Data Out"=w1290:string)  [unwired: 7 in, 2 out]
                                n327 = Unflatten From String(type=w1289, binary string=w1290) -> (value=w1287:u32)  [unwired: 3 in, 2 out]
                                n328 = Join Numbers(hi=w1288, lo=w1287) -> ()  [unwired: 1 out]
                              }
                              frame "dat", "u16" {
                                n329 = call "IMAQ ImageToArray"("error in (no error)"=w1300, "Image"=w1296) -> ("Image Pixels (I16)"=w1299:i16[][])  [unwired: 2 in, 4 out]
                                n330 = stacked-sequence {
                                seq-local: [_ _ w1306 _ _] -> [_ _ _ w1316 _]
                                tunnel: w1299 -> [_ w1304 _ _ _]
                                tunnel: w1297 -> [_ w1303 _ _ _]
                                tunnel: w1301 -> [w1302 _ _ _ w1320]
                                tunnel: w1298 -> [_ _ _ w1319 _]
                                tunnel: w1296 -> [_ _ w1307 _ _]
                                frame #0 {
                                n331 = call <vilib>:"Acquire Semaphore.vi"("semaphore"=w1302) -> ()  [unwired: 4 in, 3 out]
                                }
                                frame #1 {
                                n332 = Write to Binary File(file (use dialog)=w1303, data=w1304, 5:FALSE ("prepend array or string size? (T)")) -> ()  [unwired: 3 in, 3 out]
                                }
                                frame #2 {
                                w1310 = u32 0
                                n333 = call "IMAQ Read Custom Data"("Key"="IMAQdxReceiveTimestampHigh", "Image"=w1307) -> ("Custom Data Out"=w1314:string, "Image (duplicate)"=w1313:T4)  [unwired: 7 in, 1 out]
                                n334 = Unflatten From String(type=w1310, binary string=w1314) -> (value=w1309:u32)  [unwired: 3 in, 2 out]
                                n335 = call "IMAQ Read Custom Data"("Key"="IMAQdxReceiveTimestampLow", "Image"=w1313) -> ("Custom Data Out"=w1311:string)  [unwired: 7 in, 2 out]
                                n336 = Unflatten From String(type=w1310, binary string=w1311) -> (value=w1308:u32)  [unwired: 3 in, 2 out]
                                n337 = Join Numbers(hi=w1309, lo=w1308) -> ((hi.lo)=w1306:u64)
                                }
                                frame #3 {
                                n338 = Bundle("element"=enum16{"Camera 1", "Camera 2", "Camera 3"}."Camera 2", w1316) -> (w1318:T24)  [unwired: 1 in]
                                n339 = Enqueue Element(queue=w1319, element=w1318) -> ()  [unwired: 2 in, 3 out]
                                }
                                frame #4 {
                                n340 = call <vilib>:"Release Semaphore.vi"("semaphore"=w1320) -> ()  [unwired: 5 in, 2 out]
                                }
                                }
                              }
                            }
                            n341 = case shown="False" w1229 {
                              tunnel: w1247 -> [w1326 _]
                              tunnel: w1240 -> [w1327 _]
                              tunnel: w1242 -> [w1325 _]
                              tunnel: w1223 -> [w1324 _]
                              tunnel: w1222 -> [w1321 _]
                              tunnel: w1220 -> [w1323 _]
                              tunnel: w1219 -> [w1322 _]
                              frame False {
                                n342 = case shown="2" w1327 {
                                tunnel: w1326 -> [_ _ w1388]
                                tunnel: w1325 -> [_ _ w1387]
                                tunnel: w1324 -> [_ w1331 w1384]
                                tunnel: w1323 -> [_ w1330 _]
                                tunnel: w1322 -> [_ w1329 _]
                                tunnel: w1321 -> [_ w1328 w1383]
                                frame -1, Default {
                                }
                                frame 0 {
                                n343 = case shown="\"Anticlockwise, Flip UD\"" w1328 {
                                tunnel: w1331 -> [w1338 w1341 w1344 w1347 w1354 w1361 w1364 w1373 w1380]
                                tunnel: [w1338 w1340 w1343 w1345 w1350 w1357 w1365 w1369 w1376] -> w1332
                                frame "No rotation, No flip", Default {
                                }
                                frame "No rotation, Flip UD" {
                                w1339 = u32 0 items=["Horizontal", "Vertical", "Central", "1st Diagonal", "2nd Diagonal"] ("Type of Symmetry")
                                n344 = call "IMAQ Symmetry"("Type of Symmetry"=w1339, "Image Dst"=w1341, "Image Src"=w1341) -> ("Image Dst Out"=w1340:T4)  [unwired: 2 in, 1 out]
                                }
                                frame "No rotation, Flip LR" {
                                w1342 = u32 1 items=["Horizontal", "Vertical", "Central", "1st Diagonal", "2nd Diagonal"] ("Type of Symmetry")
                                n345 = call "IMAQ Symmetry"("Type of Symmetry"=w1342, "Image Dst"=w1344, "Image Src"=w1344) -> ("Image Dst Out"=w1343:T4)  [unwired: 2 in, 1 out]
                                }
                                frame "Clockwise, No flip" {
                                n346 = call "IMAQ Rotate"("Use Bilinear Interpolation"=FALSE, "Maintain Size"=FALSE, "Angle (degrees)"=sgl 270.0, "Image Dst"=w1347, "Image Src"=w1347) -> ("Image Dst Out"=w1345:T4)  [unwired: 5 in, 1 out]
                                }
                                frame "Clockwise, Flip UD" {
                                w1352 = u32 0 items=["Horizontal", "Vertical", "Central", "1st Diagonal", "2nd Diagonal"] ("Type of Symmetry")
                                n347 = call "IMAQ Rotate"("Use Bilinear Interpolation"=FALSE, "Maintain Size"=FALSE, "Angle (degrees)"=sgl 270.0, "Image Dst"=w1354, "Image Src"=w1354) -> ("Image Dst Out"=w1351:T4)  [unwired: 5 in, 1 out]
                                n348 = call "IMAQ Symmetry"("Type of Symmetry"=w1352, "Image Dst"=w1351, "Image Src"=w1351) -> ("Image Dst Out"=w1350:T4)  [unwired: 2 in, 1 out]
                                }
                                frame "Clockwise, Flip LR" {
                                w1359 = u32 1 items=["Horizontal", "Vertical", "Central", "1st Diagonal", "2nd Diagonal"] ("Type of Symmetry")
                                n349 = call "IMAQ Rotate"("Use Bilinear Interpolation"=FALSE, "Maintain Size"=FALSE, "Angle (degrees)"=sgl 270.0, "Image Dst"=w1361, "Image Src"=w1361) -> ("Image Dst Out"=w1358:T4)  [unwired: 5 in, 1 out]
                                n350 = call "IMAQ Symmetry"("Type of Symmetry"=w1359, "Image Dst"=w1358, "Image Src"=w1358) -> ("Image Dst Out"=w1357:T4)  [unwired: 2 in, 1 out]
                                }
                                frame "Anticlockwise, No flip" {
                                n351 = call "IMAQ Rotate"("Use Bilinear Interpolation"=FALSE, "Maintain Size"=FALSE, "Angle (degrees)"=sgl 90.0, "Image Dst"=w1364, "Image Src"=w1364) -> ("Image Dst Out"=w1365:T4)  [unwired: 5 in, 1 out]
                                }
                                frame "Anticlockwise, Flip UD" {
                                w1371 = u32 0 items=["Horizontal", "Vertical", "Central", "1st Diagonal", "2nd Diagonal"] ("Type of Symmetry")
                                n352 = call "IMAQ Rotate"("Use Bilinear Interpolation"=FALSE, "Maintain Size"=FALSE, "Angle (degrees)"=sgl 90.0, "Image Dst"=w1373, "Image Src"=w1373) -> ("Image Dst Out"=w1370:T4)  [unwired: 5 in, 1 out]
                                n353 = call "IMAQ Symmetry"("Type of Symmetry"=w1371, "Image Dst"=w1370, "Image Src"=w1370) -> ("Image Dst Out"=w1369:T4)  [unwired: 2 in, 1 out]
                                }
                                frame "Anticlockwise, Flip LR" {
                                w1378 = u32 1 items=["Horizontal", "Vertical", "Central", "1st Diagonal", "2nd Diagonal"] ("Type of Symmetry")
                                n354 = call "IMAQ Rotate"("Use Bilinear Interpolation"=FALSE, "Maintain Size"=FALSE, "Angle (degrees)"=sgl 90.0, "Image Dst"=w1380, "Image Src"=w1380) -> ("Image Dst Out"=w1377:T4)  [unwired: 5 in, 1 out]
                                n355 = call "IMAQ Symmetry"("Type of Symmetry"=w1378, "Image Dst"=w1377, "Image Src"=w1377) -> ("Image Dst Out"=w1376:T4)  [unwired: 2 in, 1 out]
                                }
                                }
                                n356 = for {
                                tunnel: w1332 -> [w1335]
                                tunnel: w1330 -> [w1334] mode=indexing
                                tunnel: w1329 -> [w1333] mode=indexing
                                n357 = case shown="\"Camera 2\"" w1334 {
                                tunnel: w1335 -> [_ w1337]
                                tunnel: w1333 -> [_ w1336]
                                frame "None", Default {
                                }
                                frame "Camera 2" {
                                n358 = call "IMAQ Copy"("Image Dst"=w1336, "Image Src"=w1337) -> ()  [unwired: 4 in, 2 out]
                                }
                                }
                                }
                                }
                                frame 2 {
                                n359 = case shown="\"Anticlockwise, Flip UD\"" w1383 {
                                tunnel: w1384 -> [w1389 w1392 w1395 w1398 w1405 w1412 w1415 w1424 w1431]
                                tunnel: [w1389 w1391 w1394 w1396 w1401 w1408 w1416 w1420 w1427] -> w1385
                                frame "No rotation, No flip", Default {
                                }
                                frame "No rotation, Flip UD" {
                                w1390 = u32 0 items=["Horizontal", "Vertical", "Central", "1st Diagonal", "2nd Diagonal"] ("Type of Symmetry")
                                n360 = call "IMAQ Symmetry"("Type of Symmetry"=w1390, "Image Dst"=w1392, "Image Src"=w1392) -> ("Image Dst Out"=w1391:T4)  [unwired: 2 in, 1 out]
                                }
                                frame "No rotation, Flip LR" {
                                w1393 = u32 1 items=["Horizontal", "Vertical", "Central", "1st Diagonal", "2nd Diagonal"] ("Type of Symmetry")
                                n361 = call "IMAQ Symmetry"("Type of Symmetry"=w1393, "Image Dst"=w1395, "Image Src"=w1395) -> ("Image Dst Out"=w1394:T4)  [unwired: 2 in, 1 out]
                                }
                                frame "Clockwise, No flip" {
                                n362 = call "IMAQ Rotate"("Use Bilinear Interpolation"=FALSE, "Maintain Size"=FALSE, "Angle (degrees)"=sgl 270.0, "Image Dst"=w1398, "Image Src"=w1398) -> ("Image Dst Out"=w1396:T4)  [unwired: 5 in, 1 out]
                                }
                                frame "Clockwise, Flip UD" {
                                w1403 = u32 0 items=["Horizontal", "Vertical", "Central", "1st Diagonal", "2nd Diagonal"] ("Type of Symmetry")
                                n363 = call "IMAQ Rotate"("Use Bilinear Interpolation"=FALSE, "Maintain Size"=FALSE, "Angle (degrees)"=sgl 270.0, "Image Dst"=w1405, "Image Src"=w1405) -> ("Image Dst Out"=w1402:T4)  [unwired: 5 in, 1 out]
                                n364 = call "IMAQ Symmetry"("Type of Symmetry"=w1403, "Image Dst"=w1402, "Image Src"=w1402) -> ("Image Dst Out"=w1401:T4)  [unwired: 2 in, 1 out]
                                }
                                frame "Clockwise, Flip LR" {
                                w1410 = u32 1 items=["Horizontal", "Vertical", "Central", "1st Diagonal", "2nd Diagonal"] ("Type of Symmetry")
                                n365 = call "IMAQ Rotate"("Use Bilinear Interpolation"=FALSE, "Maintain Size"=FALSE, "Angle (degrees)"=sgl 270.0, "Image Dst"=w1412, "Image Src"=w1412) -> ("Image Dst Out"=w1409:T4)  [unwired: 5 in, 1 out]
                                n366 = call "IMAQ Symmetry"("Type of Symmetry"=w1410, "Image Dst"=w1409, "Image Src"=w1409) -> ("Image Dst Out"=w1408:T4)  [unwired: 2 in, 1 out]
                                }
                                frame "Anticlockwise, No flip" {
                                n367 = call "IMAQ Rotate"("Use Bilinear Interpolation"=FALSE, "Maintain Size"=FALSE, "Angle (degrees)"=sgl 90.0, "Image Dst"=w1415, "Image Src"=w1415) -> ("Image Dst Out"=w1416:T4)  [unwired: 5 in, 1 out]
                                }
                                frame "Anticlockwise, Flip UD" {
                                w1422 = u32 0 items=["Horizontal", "Vertical", "Central", "1st Diagonal", "2nd Diagonal"] ("Type of Symmetry")
                                n368 = call "IMAQ Rotate"("Use Bilinear Interpolation"=FALSE, "Maintain Size"=FALSE, "Angle (degrees)"=sgl 90.0, "Image Dst"=w1424, "Image Src"=w1424) -> ("Image Dst Out"=w1421:T4)  [unwired: 5 in, 1 out]
                                n369 = call "IMAQ Symmetry"("Type of Symmetry"=w1422, "Image Dst"=w1421, "Image Src"=w1421) -> ("Image Dst Out"=w1420:T4)  [unwired: 2 in, 1 out]
                                }
                                frame "Anticlockwise, Flip LR" {
                                w1429 = u32 1 items=["Horizontal", "Vertical", "Central", "1st Diagonal", "2nd Diagonal"] ("Type of Symmetry")
                                n370 = call "IMAQ Rotate"("Use Bilinear Interpolation"=FALSE, "Maintain Size"=FALSE, "Angle (degrees)"=sgl 90.0, "Image Dst"=w1431, "Image Src"=w1431) -> ("Image Dst Out"=w1428:T4)  [unwired: 5 in, 1 out]
                                n371 = call "IMAQ Symmetry"("Type of Symmetry"=w1429, "Image Dst"=w1428, "Image Src"=w1428) -> ("Image Dst Out"=w1427:T4)  [unwired: 2 in, 1 out]
                                }
                                }
                                n372 = call "IMAQ Copy"("Image Dst"=w1388, "Image Src"=w1385) -> ("Image Dst Out"=w1386:T4)  [unwired: 4 in, 1 out]
                                n373 = property class="ImageControl"(reference=w1387, "Value"=w1386) -> ()  [unwired: 1 in, 2 out]
                                }
                                }
                              }
                              frame True {
                              }
                            }
                            n374 = property class="Bool (strict)"(reference=w1233) -> ("Value"=w1236:bool)  [unwired: 1 in, 2 out]
                            n375 = Not(x=w1236) -> (.not. x?=w1235:bool)
                          }
                        }
                      }
                    }
                    frame True {
                    }
                  }
                  n376 = case shown="False" w879 {
                    tunnel: w866 -> [w930 _]
                    tunnel: w870 -> [w929 _]
                    tunnel: w869 -> [w928 _]
                    tunnel: w873 -> [w927 _]
                    tunnel: w874 -> [w926 _]
                    tunnel: w875 -> [w925 _]
                    tunnel: w876 -> [w924 _]
                    tunnel: w877 -> [w923 _]
                    tunnel: w871 -> [w922 _]
                    tunnel: w868 -> [w921 _]
                    tunnel: w864 -> [w920 _]
                    tunnel: w863 -> [w919 _]
                    tunnel: w862 -> [w918 _]
                    tunnel: w861 -> [w917 _]
                    tunnel: w878 -> [w916 _]
                    tunnel: w872 -> [w915 _]
                    tunnel: w859 -> [w914 _]
                    tunnel: w865 -> [w913 _]
                    tunnel: w860 -> [w912 _]
                    tunnel: w867 -> [w910 _]
                    frame False {
                      n377 = for {
                        N: w927 -> [_]
                        tunnel: w921 -> [w951]
                        tunnel: w919 -> [w950]
                        tunnel: w930 -> [w949]
                        tunnel: w928 -> [w948]
                        tunnel: w929 -> [w947]
                        tunnel: w920 -> [w946]
                        tunnel: w925 -> [w944]
                        tunnel: w926 -> [w943]
                        tunnel: w924 -> [w942]
                        tunnel: w923 -> [w941]
                        tunnel: w918 -> [w940]
                        tunnel: w922 -> [w939]
                        tunnel: w917 -> [w938]
                        tunnel: w916 -> [w937]
                        tunnel: w915 -> [w936]
                        tunnel: w914 -> [w935]
                        border: u32 0 ("millisecond timer value") -> [_]
                        tunnel: w913 -> [w933]
                        tunnel: w912 -> [w932]
                        tunnel: w910 -> [w931]
                        stop <- w934 stop-if-true
                        n378 = event shown="[1] <Session Out>: Frame Done" {
                          selector: w949 -> [_ _]
                          dyn-events: _ -> [_ _]
                          timeout: 1000 -> [_ _]
                          tunnel: w951 -> [_ _]
                          tunnel: w950 -> [_ w985]
                          tunnel: w948 -> [_ w979]
                          tunnel: w947 -> [_ w975]
                          tunnel: w946 -> [_ w978]
                          tunnel: w944 -> [_ w983]
                          tunnel: w943 -> [_ w955]
                          tunnel: w942 -> [_ w982]
                          tunnel: w941 -> [_ w981]
                          tunnel: w940 -> [_ w980]
                          tunnel: w939 -> [_ w976]
                          tunnel: w938 -> [_ w972]
                          tunnel: w937 -> [_ w977]
                          tunnel: w936 -> [_ w960]
                          tunnel: w935 -> [w954 w971]
                          tunnel: [w952 w973] -> w934
                          tunnel: w933 -> [_ w958]
                          tunnel: w932 -> [_ w957]
                          tunnel: w931 -> [_ w956]
                          event Timeout {
                            n379 = event-data() -> ()  [unwired: 1 in, 3 out]
                            n380 = property class="Bool (strict)"(reference=w954) -> ("Value"=w953:bool)  [unwired: 1 in, 2 out]
                            n381 = Not(x=w953) -> (.not. x?=w952:bool)
                          }
                          event event #0x0 {
                            # "Read data"
                            n382 = event-data() -> ()  [unwired: 1 in, 1 out]
                            n383 = Tick Count (ms)() -> (millisecond timer value=w959:u32)
                            n384 = feedback #4() -> (w968:u32)
                            n385 = call "Elapsed time.vi"("Start time (ms)"=w968, "Current time (ms)"=w959) -> ("Elapsed time"=w970:u32)
                            n386 = Greater?(x=w970, y=w956) -> (0:w964:bool)
                            n387 = Select(t=w959, s=w964, f=w968) -> (s? t:f=w969:u32)
                            n388 = feedback-in #4(w969) -> ()
                            n389 = call <vilib>:"IMAQdx Get Image2.vi"("Buffer Number Mode (Next)"=IMAQdx_Buffer_Number_Mode."Last New", "Image In"=w975, "Session In"=w979) -> ("error out"=w962:errorcluster, "Image Out"=w963:T4)  [unwired: 5 in, 2 out]
                            n390 = Not A Number/Path/Refnum?(number/path/refnum=w985) -> (NaN/Path/Refnum?=w966:bool)
                            n391 = Not(x=w964) -> (.not. x?=w965:bool)
                            n392 = Or(x=w966, y=w965) -> (x .or. y?=w967:bool)
                            n393 = case shown="\"'tiff'\", \"tif\"" w955 {
                              tunnel: w963 -> [w987 w1031 w1034]
                              tunnel: w983 -> [_ _ w1035]
                              tunnel: w982 -> [w988 _ _]
                              tunnel: w981 -> [w989 _ _]
                              tunnel: w976 -> [w993 _ _]
                              tunnel: w972 -> [w992 _ w1039]
                              tunnel: w977 -> [w991 _ w1036]
                              tunnel: w962 -> [w990 _ w1038]
                              tunnel: [w986 w1031 w1034] -> w961
                              frame "'tiff'", "tif" {
                                n394 = stacked-sequence {
                                tunnel: w993 -> [_ w1007 _ _]
                                tunnel: w992 -> [w994 _ _ w1024]
                                tunnel: w991 -> [_ _ w1022 _]
                                tunnel: w990 -> [_ w1002 _ _]
                                tunnel: w989 -> [_ w1001 _ _]
                                tunnel: w988 -> [_ w997 _ _]
                                tunnel: w987 -> [_ w999 w1013 _]
                                tunnel: [_ w999 _ _] -> w986
                                frame #0 {
                                n395 = call <vilib>:"Acquire Semaphore.vi"("semaphore"=w994) -> ()  [unwired: 4 in, 3 out]
                                }
                                frame #1 {
                                n396 = Preview Queue Element(queue=w997) -> (queue out=w998:refnum<queue>, element=w996:T11)  [unwired: 2 in, 2 out]
                                n397 = in-place {
                                in-place-border: w999 -> [w1010]
                                in-place-border: w1002 -> [w1009]
                                n398 = in-place-dvr #5(w1001) -> ()  [unwired: 2 out]
                                n399 = call "IMAQ ImageToArray"("error in (no error)"=w1009, "Image"=w1010) -> ("Image Pixels (I16)"=w1008:i16[][])  [unwired: 2 in, 4 out]
                                n400 = in-place-dvr #5(w1008) -> (w1000:refnum<data-value>)  [unwired: 1 out]
                                }
                                n401 = Preview Queue Element(queue=w1007) -> (queue out=w1005:refnum<queue>, element=w1006:u32[])  [unwired: 2 in, 2 out]
                                n402 = call "TIFFStream Write.vi"("File data"=w996, "Last image in file?"=FALSE, "Current and next IFD offset in"=w1006, "Image data reference"=w1000) -> ("Current and next IFD offset out"=w1004:u32[], "File data out"=w995:T11)  [unwired: 5 in, 1 out]
                                n403 = Lossy Enqueue Element(queue=w998, element=w995) -> ()  [unwired: 1 in, 4 out]
                                n404 = Lossy Enqueue Element(queue=w1005, element=w1004) -> ()  [unwired: 1 in, 4 out]
                                }
                                frame #2 {
                                w1016 = u32 0
                                n405 = call "IMAQ Read Custom Data"("Key"="IMAQdxReceiveTimestampHigh", "Image"=w1013) -> ("Custom Data Out"=w1020:string, "Image (duplicate)"=w1019:T4)  [unwired: 7 in, 1 out]
                                n406 = Unflatten From String(type=w1016, binary string=w1020) -> (value=w1015:u32)  [unwired: 3 in, 2 out]
                                n407 = call "IMAQ Read Custom Data"("Key"="IMAQdxReceiveTimestampLow", "Image"=w1019) -> ("Custom Data Out"=w1017:string)  [unwired: 7 in, 2 out]
                                n408 = Unflatten From String(type=w1016, binary string=w1017) -> (value=w1014:u32)  [unwired: 3 in, 2 out]
                                n409 = Join Numbers(hi=w1015, lo=w1014) -> ((hi.lo)=w1011:u64)
                                n410 = Bundle("element"=enum16{"Camera 1", "Camera 2", "Camera 3"}."Camera 3", w1011) -> (w1012:T24)  [unwired: 1 in]
                                n411 = Enqueue Element(queue=w1022, element=w1012) -> ()  [unwired: 2 in, 3 out]
                                }
                                frame #3 {
                                n412 = call <vilib>:"Release Semaphore.vi"("semaphore"=w1024) -> ()  [unwired: 5 in, 2 out]
                                }
                                }
                              }
                              frame "None", Default {
                                w1027 = u32 0
                                n413 = call "IMAQ Read Custom Data"("Key"="IMAQdxReceiveTimestampHigh", "Image"=w1031) -> ("Custom Data Out"=w1032:string, "Image (duplicate)"=w1030:T4)  [unwired: 7 in, 1 out]
                                n414 = Unflatten From String(type=w1027, binary string=w1032) -> (value=w1026:u32)  [unwired: 3 in, 2 out]
                                n415 = call "IMAQ Read Custom Data"("Key"="IMAQdxReceiveTimestampLow", "Image"=w1030) -> ("Custom Data Out"=w1028:string)  [unwired: 7 in, 2 out]
                                n416 = Unflatten From String(type=w1027, binary string=w1028) -> (value=w1025:u32)  [unwired: 3 in, 2 out]
                                n417 = Join Numbers(hi=w1026, lo=w1025) -> ()  [unwired: 1 out]
                              }
                              frame "dat", "u16" {
                                n418 = call "IMAQ ImageToArray"("error in (no error)"=w1038, "Image"=w1034) -> ("Image Pixels (I16)"=w1037:i16[][])  [unwired: 2 in, 4 out]
                                n419 = stacked-sequence {
                                seq-local: [_ _ w1044 _ _] -> [_ _ _ w1054 _]
                                tunnel: w1037 -> [_ w1042 _ _ _]
                                tunnel: w1035 -> [_ w1041 _ _ _]
                                tunnel: w1039 -> [w1040 _ _ _ w1058]
                                tunnel: w1036 -> [_ _ _ w1057 _]
                                tunnel: w1034 -> [_ _ w1045 _ _]
                                frame #0 {
                                n420 = call <vilib>:"Acquire Semaphore.vi"("semaphore"=w1040) -> ()  [unwired: 4 in, 3 out]
                                }
                                frame #1 {
                                n421 = Write to Binary File(file (use dialog)=w1041, data=w1042, 5:FALSE ("prepend array or string size? (T)")) -> ()  [unwired: 3 in, 3 out]
                                }
                                frame #2 {
                                w1048 = u32 0
                                n422 = call "IMAQ Read Custom Data"("Key"="IMAQdxReceiveTimestampHigh", "Image"=w1045) -> ("Custom Data Out"=w1052:string, "Image (duplicate)"=w1051:T4)  [unwired: 7 in, 1 out]
                                n423 = Unflatten From String(type=w1048, binary string=w1052) -> (value=w1047:u32)  [unwired: 3 in, 2 out]
                                n424 = call "IMAQ Read Custom Data"("Key"="IMAQdxReceiveTimestampLow", "Image"=w1051) -> ("Custom Data Out"=w1049:string)  [unwired: 7 in, 2 out]
                                n425 = Unflatten From String(type=w1048, binary string=w1049) -> (value=w1046:u32)  [unwired: 3 in, 2 out]
                                n426 = Join Numbers(hi=w1047, lo=w1046) -> ((hi.lo)=w1044:u64)
                                }
                                frame #3 {
                                n427 = Bundle("element"=enum16{"Camera 1", "Camera 2", "Camera 3"}."Camera 3", w1054) -> (w1056:T24)  [unwired: 1 in]
                                n428 = Enqueue Element(queue=w1057, element=w1056) -> ()  [unwired: 2 in, 3 out]
                                }
                                frame #4 {
                                n429 = call <vilib>:"Release Semaphore.vi"("semaphore"=w1058) -> ()  [unwired: 5 in, 2 out]
                                }
                                }
                              }
                            }
                            n430 = case shown="False" w967 {
                              tunnel: w985 -> [w1064 _]
                              tunnel: w978 -> [w1065 _]
                              tunnel: w980 -> [w1063 _]
                              tunnel: w961 -> [w1062 _]
                              tunnel: w960 -> [w1059 _]
                              tunnel: w958 -> [w1061 _]
                              tunnel: w957 -> [w1060 _]
                              frame False {
                                n431 = case shown="0" w1065 {
                                tunnel: w1064 -> [_ _ w1126]
                                tunnel: w1063 -> [_ _ w1125]
                                tunnel: w1062 -> [_ w1069 w1122]
                                tunnel: w1061 -> [_ w1068 _]
                                tunnel: w1060 -> [_ w1067 _]
                                tunnel: w1059 -> [_ w1066 w1121]
                                frame -1, Default {
                                }
                                frame 0 {
                                n432 = case shown="\"Anticlockwise, Flip UD\"" w1066 {
                                tunnel: w1069 -> [w1076 w1079 w1082 w1085 w1092 w1099 w1102 w1111 w1118]
                                tunnel: [w1076 w1078 w1081 w1083 w1088 w1095 w1103 w1107 w1114] -> w1070
                                frame "No rotation, No flip", Default {
                                }
                                frame "No rotation, Flip UD" {
                                w1077 = u32 0 items=["Horizontal", "Vertical", "Central", "1st Diagonal", "2nd Diagonal"] ("Type of Symmetry")
                                n433 = call "IMAQ Symmetry"("Type of Symmetry"=w1077, "Image Dst"=w1079, "Image Src"=w1079) -> ("Image Dst Out"=w1078:T4)  [unwired: 2 in, 1 out]
                                }
                                frame "No rotation, Flip LR" {
                                w1080 = u32 1 items=["Horizontal", "Vertical", "Central", "1st Diagonal", "2nd Diagonal"] ("Type of Symmetry")
                                n434 = call "IMAQ Symmetry"("Type of Symmetry"=w1080, "Image Dst"=w1082, "Image Src"=w1082) -> ("Image Dst Out"=w1081:T4)  [unwired: 2 in, 1 out]
                                }
                                frame "Clockwise, No flip" {
                                n435 = call "IMAQ Rotate"("Use Bilinear Interpolation"=FALSE, "Maintain Size"=FALSE, "Angle (degrees)"=sgl 270.0, "Image Dst"=w1085, "Image Src"=w1085) -> ("Image Dst Out"=w1083:T4)  [unwired: 5 in, 1 out]
                                }
                                frame "Clockwise, Flip UD" {
                                w1090 = u32 0 items=["Horizontal", "Vertical", "Central", "1st Diagonal", "2nd Diagonal"] ("Type of Symmetry")
                                n436 = call "IMAQ Rotate"("Use Bilinear Interpolation"=FALSE, "Maintain Size"=FALSE, "Angle (degrees)"=sgl 270.0, "Image Dst"=w1092, "Image Src"=w1092) -> ("Image Dst Out"=w1089:T4)  [unwired: 5 in, 1 out]
                                n437 = call "IMAQ Symmetry"("Type of Symmetry"=w1090, "Image Dst"=w1089, "Image Src"=w1089) -> ("Image Dst Out"=w1088:T4)  [unwired: 2 in, 1 out]
                                }
                                frame "Clockwise, Flip LR" {
                                w1097 = u32 1 items=["Horizontal", "Vertical", "Central", "1st Diagonal", "2nd Diagonal"] ("Type of Symmetry")
                                n438 = call "IMAQ Rotate"("Use Bilinear Interpolation"=FALSE, "Maintain Size"=FALSE, "Angle (degrees)"=sgl 270.0, "Image Dst"=w1099, "Image Src"=w1099) -> ("Image Dst Out"=w1096:T4)  [unwired: 5 in, 1 out]
                                n439 = call "IMAQ Symmetry"("Type of Symmetry"=w1097, "Image Dst"=w1096, "Image Src"=w1096) -> ("Image Dst Out"=w1095:T4)  [unwired: 2 in, 1 out]
                                }
                                frame "Anticlockwise, No flip" {
                                n440 = call "IMAQ Rotate"("Use Bilinear Interpolation"=FALSE, "Maintain Size"=FALSE, "Angle (degrees)"=sgl 90.0, "Image Dst"=w1102, "Image Src"=w1102) -> ("Image Dst Out"=w1103:T4)  [unwired: 5 in, 1 out]
                                }
                                frame "Anticlockwise, Flip UD" {
                                w1109 = u32 0 items=["Horizontal", "Vertical", "Central", "1st Diagonal", "2nd Diagonal"] ("Type of Symmetry")
                                n441 = call "IMAQ Rotate"("Use Bilinear Interpolation"=FALSE, "Maintain Size"=FALSE, "Angle (degrees)"=sgl 90.0, "Image Dst"=w1111, "Image Src"=w1111) -> ("Image Dst Out"=w1108:T4)  [unwired: 5 in, 1 out]
                                n442 = call "IMAQ Symmetry"("Type of Symmetry"=w1109, "Image Dst"=w1108, "Image Src"=w1108) -> ("Image Dst Out"=w1107:T4)  [unwired: 2 in, 1 out]
                                }
                                frame "Anticlockwise, Flip LR" {
                                w1116 = u32 1 items=["Horizontal", "Vertical", "Central", "1st Diagonal", "2nd Diagonal"] ("Type of Symmetry")
                                n443 = call "IMAQ Rotate"("Use Bilinear Interpolation"=FALSE, "Maintain Size"=FALSE, "Angle (degrees)"=sgl 90.0, "Image Dst"=w1118, "Image Src"=w1118) -> ("Image Dst Out"=w1115:T4)  [unwired: 5 in, 1 out]
                                n444 = call "IMAQ Symmetry"("Type of Symmetry"=w1116, "Image Dst"=w1115, "Image Src"=w1115) -> ("Image Dst Out"=w1114:T4)  [unwired: 2 in, 1 out]
                                }
                                }
                                n445 = for {
                                tunnel: w1070 -> [w1073]
                                tunnel: w1068 -> [w1072] mode=indexing
                                tunnel: w1067 -> [w1071] mode=indexing
                                n446 = case shown="\"Camera 3\"" w1072 {
                                tunnel: w1073 -> [_ w1075]
                                tunnel: w1071 -> [_ w1074]
                                frame "None", Default {
                                }
                                frame "Camera 3" {
                                n447 = call "IMAQ Copy"("Image Dst"=w1074, "Image Src"=w1075) -> ()  [unwired: 4 in, 2 out]
                                }
                                }
                                }
                                }
                                frame 3 {
                                n448 = case shown="\"Anticlockwise, Flip UD\"" w1121 {
                                tunnel: w1122 -> [w1127 w1130 w1133 w1136 w1143 w1150 w1153 w1162 w1169]
                                tunnel: [w1127 w1129 w1132 w1134 w1139 w1146 w1154 w1158 w1165] -> w1123
                                frame "No rotation, No flip", Default {
                                }
                                frame "No rotation, Flip UD" {
                                w1128 = u32 0 items=["Horizontal", "Vertical", "Central", "1st Diagonal", "2nd Diagonal"] ("Type of Symmetry")
                                n449 = call "IMAQ Symmetry"("Type of Symmetry"=w1128, "Image Dst"=w1130, "Image Src"=w1130) -> ("Image Dst Out"=w1129:T4)  [unwired: 2 in, 1 out]
                                }
                                frame "No rotation, Flip LR" {
                                w1131 = u32 1 items=["Horizontal", "Vertical", "Central", "1st Diagonal", "2nd Diagonal"] ("Type of Symmetry")
                                n450 = call "IMAQ Symmetry"("Type of Symmetry"=w1131, "Image Dst"=w1133, "Image Src"=w1133) -> ("Image Dst Out"=w1132:T4)  [unwired: 2 in, 1 out]
                                }
                                frame "Clockwise, No flip" {
                                n451 = call "IMAQ Rotate"("Use Bilinear Interpolation"=FALSE, "Maintain Size"=FALSE, "Angle (degrees)"=sgl 270.0, "Image Dst"=w1136, "Image Src"=w1136) -> ("Image Dst Out"=w1134:T4)  [unwired: 5 in, 1 out]
                                }
                                frame "Clockwise, Flip UD" {
                                w1141 = u32 0 items=["Horizontal", "Vertical", "Central", "1st Diagonal", "2nd Diagonal"] ("Type of Symmetry")
                                n452 = call "IMAQ Rotate"("Use Bilinear Interpolation"=FALSE, "Maintain Size"=FALSE, "Angle (degrees)"=sgl 270.0, "Image Dst"=w1143, "Image Src"=w1143) -> ("Image Dst Out"=w1140:T4)  [unwired: 5 in, 1 out]
                                n453 = call "IMAQ Symmetry"("Type of Symmetry"=w1141, "Image Dst"=w1140, "Image Src"=w1140) -> ("Image Dst Out"=w1139:T4)  [unwired: 2 in, 1 out]
                                }
                                frame "Clockwise, Flip LR" {
                                w1148 = u32 1 items=["Horizontal", "Vertical", "Central", "1st Diagonal", "2nd Diagonal"] ("Type of Symmetry")
                                n454 = call "IMAQ Rotate"("Use Bilinear Interpolation"=FALSE, "Maintain Size"=FALSE, "Angle (degrees)"=sgl 270.0, "Image Dst"=w1150, "Image Src"=w1150) -> ("Image Dst Out"=w1147:T4)  [unwired: 5 in, 1 out]
                                n455 = call "IMAQ Symmetry"("Type of Symmetry"=w1148, "Image Dst"=w1147, "Image Src"=w1147) -> ("Image Dst Out"=w1146:T4)  [unwired: 2 in, 1 out]
                                }
                                frame "Anticlockwise, No flip" {
                                n456 = call "IMAQ Rotate"("Use Bilinear Interpolation"=FALSE, "Maintain Size"=FALSE, "Angle (degrees)"=sgl 90.0, "Image Dst"=w1153, "Image Src"=w1153) -> ("Image Dst Out"=w1154:T4)  [unwired: 5 in, 1 out]
                                }
                                frame "Anticlockwise, Flip UD" {
                                w1160 = u32 0 items=["Horizontal", "Vertical", "Central", "1st Diagonal", "2nd Diagonal"] ("Type of Symmetry")
                                n457 = call "IMAQ Rotate"("Use Bilinear Interpolation"=FALSE, "Maintain Size"=FALSE, "Angle (degrees)"=sgl 90.0, "Image Dst"=w1162, "Image Src"=w1162) -> ("Image Dst Out"=w1159:T4)  [unwired: 5 in, 1 out]
                                n458 = call "IMAQ Symmetry"("Type of Symmetry"=w1160, "Image Dst"=w1159, "Image Src"=w1159) -> ("Image Dst Out"=w1158:T4)  [unwired: 2 in, 1 out]
                                }
                                frame "Anticlockwise, Flip LR" {
                                w1167 = u32 1 items=["Horizontal", "Vertical", "Central", "1st Diagonal", "2nd Diagonal"] ("Type of Symmetry")
                                n459 = call "IMAQ Rotate"("Use Bilinear Interpolation"=FALSE, "Maintain Size"=FALSE, "Angle (degrees)"=sgl 90.0, "Image Dst"=w1169, "Image Src"=w1169) -> ("Image Dst Out"=w1166:T4)  [unwired: 5 in, 1 out]
                                n460 = call "IMAQ Symmetry"("Type of Symmetry"=w1167, "Image Dst"=w1166, "Image Src"=w1166) -> ("Image Dst Out"=w1165:T4)  [unwired: 2 in, 1 out]
                                }
                                }
                                n461 = call "IMAQ Copy"("Image Dst"=w1126, "Image Src"=w1123) -> ("Image Dst Out"=w1124:T4)  [unwired: 4 in, 1 out]
                                n462 = property class="ImageControl"(reference=w1125, "Value"=w1124) -> ()  [unwired: 1 in, 2 out]
                                }
                                }
                              }
                              frame True {
                              }
                            }
                            n463 = property class="Bool (strict)"(reference=w971) -> ("Value"=w974:bool)  [unwired: 1 in, 2 out]
                            n464 = Not(x=w974) -> (.not. x?=w973:bool)
                          }
                        }
                      }
                    }
                    frame True {
                    }
                  }
                  n465 = case shown="False" w895 {
                    tunnel: w894 -> [w1454 _]
                    tunnel: w902 -> [w1453 _]
                    tunnel: w898 -> [w1452 _]
                    tunnel: w873 -> [w1451 _]
                    tunnel: w874 -> [w1450 _]
                    tunnel: w875 -> [w1449 _]
                    tunnel: w876 -> [w1448 _]
                    tunnel: w877 -> [w1447 _]
                    tunnel: w871 -> [w1446 _]
                    tunnel: w868 -> [w1445 _]
                    tunnel: w864 -> [w1444 _]
                    tunnel: w863 -> [w1443 _]
                    tunnel: w862 -> [w1442 _]
                    tunnel: w861 -> [w1441 _]
                    tunnel: w878 -> [w1440 _]
                    tunnel: w889 -> [w1439 _]
                    tunnel: w859 -> [w1438 _]
                    tunnel: w865 -> [w1437 _]
                    tunnel: w860 -> [w1436 _]
                    tunnel: w885 -> [w1434 _]
                    frame False {
                      n466 = for {
                        N: w1451 -> [_]
                        tunnel: w1445 -> [w1475]
                        tunnel: w1443 -> [w1474]
                        tunnel: w1454 -> [w1473]
                        tunnel: w1452 -> [w1472]
                        tunnel: w1453 -> [w1471]
                        tunnel: w1444 -> [w1470]
                        tunnel: w1449 -> [w1468]
                        tunnel: w1450 -> [w1467]
                        tunnel: w1448 -> [w1466]
                        tunnel: w1447 -> [w1465]
                        tunnel: w1442 -> [w1464]
                        tunnel: w1446 -> [w1463]
                        tunnel: w1441 -> [w1462]
                        tunnel: w1440 -> [w1461]
                        tunnel: w1439 -> [w1460]
                        tunnel: w1438 -> [w1459]
                        border: u32 0 ("millisecond timer value") -> [_]
                        tunnel: w1437 -> [w1457]
                        tunnel: w1436 -> [w1456]
                        tunnel: w1434 -> [w1455]
                        stop <- w1458 stop-if-true
                        n467 = event shown="[1] <Session Out>: Frame Done" {
                          selector: w1473 -> [_ _]
                          dyn-events: _ -> [_ _]
                          timeout: 1000 -> [_ _]
                          tunnel: w1475 -> [_ _]
                          tunnel: w1474 -> [_ w1509]
                          tunnel: w1472 -> [_ w1503]
                          tunnel: w1471 -> [_ w1499]
                          tunnel: w1470 -> [_ w1502]
                          tunnel: w1468 -> [_ w1507]
                          tunnel: w1467 -> [_ w1479]
                          tunnel: w1466 -> [_ w1506]
                          tunnel: w1465 -> [_ w1505]
                          tunnel: w1464 -> [_ w1504]
                          tunnel: w1463 -> [_ w1500]
                          tunnel: w1462 -> [_ w1496]
                          tunnel: w1461 -> [_ w1501]
                          tunnel: w1460 -> [_ w1484]
                          tunnel: w1459 -> [w1478 w1495]
                          tunnel: [w1476 w1497] -> w1458
                          tunnel: w1457 -> [_ w1482]
                          tunnel: w1456 -> [_ w1481]
                          tunnel: w1455 -> [_ w1480]
                          event Timeout {
                            n468 = event-data() -> ()  [unwired: 1 in, 3 out]
                            n469 = property class="Bool (strict)"(reference=w1478) -> ("Value"=w1477:bool)  [unwired: 1 in, 2 out]
                            n470 = Not(x=w1477) -> (.not. x?=w1476:bool)
                          }
                          event event #0x0 {
                            # "Read data"
                            n471 = event-data() -> ()  [unwired: 1 in, 1 out]
                            n472 = Tick Count (ms)() -> (millisecond timer value=w1483:u32)
                            n473 = feedback #6() -> (w1492:u32)
                            n474 = call "Elapsed time.vi"("Start time (ms)"=w1492, "Current time (ms)"=w1483) -> ("Elapsed time"=w1494:u32)
                            n475 = Greater?(x=w1494, y=w1480) -> (0:w1488:bool)
                            n476 = Select(t=w1483, s=w1488, f=w1492) -> (s? t:f=w1493:u32)
                            n477 = feedback-in #6(w1493) -> ()
                            n478 = call <vilib>:"IMAQdx Get Image2.vi"("Buffer Number Mode (Next)"=IMAQdx_Buffer_Number_Mode."Last New", "Image In"=w1499, "Session In"=w1503) -> ("error out"=w1486:errorcluster, "Image Out"=w1487:T4)  [unwired: 5 in, 2 out]
                            n479 = Not A Number/Path/Refnum?(number/path/refnum=w1509) -> (NaN/Path/Refnum?=w1490:bool)
                            n480 = Not(x=w1488) -> (.not. x?=w1489:bool)
                            n481 = Or(x=w1490, y=w1489) -> (x .or. y?=w1491:bool)
                            n482 = case shown="\"'tiff'\", \"tif\"" w1479 {
                              tunnel: w1487 -> [w1511 w1555 w1558]
                              tunnel: w1507 -> [_ _ w1559]
                              tunnel: w1506 -> [w1512 _ _]
                              tunnel: w1505 -> [w1513 _ _]
                              tunnel: w1500 -> [w1517 _ _]
                              tunnel: w1496 -> [w1516 _ w1563]
                              tunnel: w1501 -> [w1515 _ w1560]
                              tunnel: w1486 -> [w1514 _ w1562]
                              tunnel: [w1510 w1555 w1558] -> w1485
                              frame "'tiff'", "tif" {
                                n483 = stacked-sequence {
                                tunnel: w1517 -> [_ w1531 _ _]
                                tunnel: w1516 -> [w1518 _ _ w1548]
                                tunnel: w1515 -> [_ _ w1546 _]
                                tunnel: w1514 -> [_ w1526 _ _]
                                tunnel: w1513 -> [_ w1525 _ _]
                                tunnel: w1512 -> [_ w1521 _ _]
                                tunnel: w1511 -> [_ w1523 w1537 _]
                                tunnel: [_ w1523 _ _] -> w1510
                                frame #0 {
                                n484 = call <vilib>:"Acquire Semaphore.vi"("semaphore"=w1518) -> ()  [unwired: 4 in, 3 out]
                                }
                                frame #1 {
                                n485 = Preview Queue Element(queue=w1521) -> (queue out=w1522:refnum<queue>, element=w1520:T11)  [unwired: 2 in, 2 out]
                                n486 = in-place {
                                in-place-border: w1523 -> [w1534]
                                in-place-border: w1526 -> [w1533]
                                n487 = in-place-dvr #7(w1525) -> ()  [unwired: 2 out]
                                n488 = call "IMAQ ImageToArray"("error in (no error)"=w1533, "Image"=w1534) -> ("Image Pixels (I16)"=w1532:i16[][])  [unwired: 2 in, 4 out]
                                n489 = in-place-dvr #7(w1532) -> (w1524:refnum<data-value>)  [unwired: 1 out]
                                }
                                n490 = Preview Queue Element(queue=w1531) -> (queue out=w1529:refnum<queue>, element=w1530:u32[])  [unwired: 2 in, 2 out]
                                n491 = call "TIFFStream Write.vi"("File data"=w1520, "Last image in file?"=FALSE, "Current and next IFD offset in"=w1530, "Image data reference"=w1524) -> ("Current and next IFD offset out"=w1528:u32[], "File data out"=w1519:T11)  [unwired: 5 in, 1 out]
                                n492 = Lossy Enqueue Element(queue=w1522, element=w1519) -> ()  [unwired: 1 in, 4 out]
                                n493 = Lossy Enqueue Element(queue=w1529, element=w1528) -> ()  [unwired: 1 in, 4 out]
                                }
                                frame #2 {
                                w1540 = u32 0
                                n494 = call "IMAQ Read Custom Data"("Key"="IMAQdxReceiveTimestampHigh", "Image"=w1537) -> ("Custom Data Out"=w1544:string, "Image (duplicate)"=w1543:T4)  [unwired: 7 in, 1 out]
                                n495 = Unflatten From String(type=w1540, binary string=w1544) -> (value=w1539:u32)  [unwired: 3 in, 2 out]
                                n496 = call "IMAQ Read Custom Data"("Key"="IMAQdxReceiveTimestampLow", "Image"=w1543) -> ("Custom Data Out"=w1541:string)  [unwired: 7 in, 2 out]
                                n497 = Unflatten From String(type=w1540, binary string=w1541) -> (value=w1538:u32)  [unwired: 3 in, 2 out]
                                n498 = Join Numbers(hi=w1539, lo=w1538) -> ((hi.lo)=w1535:u64)
                                n499 = Bundle("element"=enum16{"Camera 1", "Camera 2", "Camera 3"}."Camera 1", w1535) -> (w1536:T24)  [unwired: 1 in]
                                n500 = Enqueue Element(queue=w1546, element=w1536) -> ()  [unwired: 2 in, 3 out]
                                }
                                frame #3 {
                                n501 = call <vilib>:"Release Semaphore.vi"("semaphore"=w1548) -> ()  [unwired: 5 in, 2 out]
                                }
                                }
                              }
                              frame "None", Default {
                                w1551 = u32 0
                                n502 = call "IMAQ Read Custom Data"("Key"="IMAQdxReceiveTimestampHigh", "Image"=w1555) -> ("Custom Data Out"=w1556:string, "Image (duplicate)"=w1554:T4)  [unwired: 7 in, 1 out]
                                n503 = Unflatten From String(type=w1551, binary string=w1556) -> (value=w1550:u32)  [unwired: 3 in, 2 out]
                                n504 = call "IMAQ Read Custom Data"("Key"="IMAQdxReceiveTimestampLow", "Image"=w1554) -> ("Custom Data Out"=w1552:string)  [unwired: 7 in, 2 out]
                                n505 = Unflatten From String(type=w1551, binary string=w1552) -> (value=w1549:u32)  [unwired: 3 in, 2 out]
                                n506 = Join Numbers(hi=w1550, lo=w1549) -> ()  [unwired: 1 out]
                              }
                              frame "dat", "u16" {
                                n507 = call "IMAQ ImageToArray"("error in (no error)"=w1562, "Image"=w1558) -> ("Image Pixels (I16)"=w1561:i16[][])  [unwired: 2 in, 4 out]
                                n508 = stacked-sequence {
                                seq-local: [_ _ w1568 _ _] -> [_ _ _ w1578 _]
                                tunnel: w1561 -> [_ w1566 _ _ _]
                                tunnel: w1559 -> [_ w1565 _ _ _]
                                tunnel: w1563 -> [w1564 _ _ _ w1582]
                                tunnel: w1560 -> [_ _ _ w1581 _]
                                tunnel: w1558 -> [_ _ w1569 _ _]
                                frame #0 {
                                n509 = call <vilib>:"Acquire Semaphore.vi"("semaphore"=w1564) -> ()  [unwired: 4 in, 3 out]
                                }
                                frame #1 {
                                n510 = Write to Binary File(file (use dialog)=w1565, data=w1566, 5:FALSE ("prepend array or string size? (T)")) -> ()  [unwired: 3 in, 3 out]
                                }
                                frame #2 {
                                w1572 = u32 0
                                n511 = call "IMAQ Read Custom Data"("Key"="IMAQdxReceiveTimestampHigh", "Image"=w1569) -> ("Custom Data Out"=w1576:string, "Image (duplicate)"=w1575:T4)  [unwired: 7 in, 1 out]
                                n512 = Unflatten From String(type=w1572, binary string=w1576) -> (value=w1571:u32)  [unwired: 3 in, 2 out]
                                n513 = call "IMAQ Read Custom Data"("Key"="IMAQdxReceiveTimestampLow", "Image"=w1575) -> ("Custom Data Out"=w1573:string)  [unwired: 7 in, 2 out]
                                n514 = Unflatten From String(type=w1572, binary string=w1573) -> (value=w1570:u32)  [unwired: 3 in, 2 out]
                                n515 = Join Numbers(hi=w1571, lo=w1570) -> ((hi.lo)=w1568:u64)
                                }
                                frame #3 {
                                n516 = Bundle("element"=enum16{"Camera 1", "Camera 2", "Camera 3"}."Camera 1", w1578) -> (w1580:T24)  [unwired: 1 in]
                                n517 = Enqueue Element(queue=w1581, element=w1580) -> ()  [unwired: 2 in, 3 out]
                                }
                                frame #4 {
                                n518 = call <vilib>:"Release Semaphore.vi"("semaphore"=w1582) -> ()  [unwired: 5 in, 2 out]
                                }
                                }
                              }
                            }
                            n519 = case shown="False" w1491 {
                              tunnel: w1509 -> [w1588 _]
                              tunnel: w1502 -> [w1589 _]
                              tunnel: w1504 -> [w1587 _]
                              tunnel: w1485 -> [w1586 _]
                              tunnel: w1484 -> [w1583 _]
                              tunnel: w1482 -> [w1585 _]
                              tunnel: w1481 -> [w1584 _]
                              frame False {
                                n520 = case shown="1" w1589 {
                                tunnel: w1588 -> [_ _ w1650]
                                tunnel: w1587 -> [_ _ w1649]
                                tunnel: w1586 -> [_ w1593 w1646]
                                tunnel: w1585 -> [_ w1592 _]
                                tunnel: w1584 -> [_ w1591 _]
                                tunnel: w1583 -> [_ w1590 w1645]
                                frame -1, Default {
                                }
                                frame 0 {
                                n521 = case shown="\"Anticlockwise, Flip UD\"" w1590 {
                                tunnel: w1593 -> [w1600 w1603 w1606 w1609 w1616 w1623 w1626 w1635 w1642]
                                tunnel: [w1600 w1602 w1605 w1607 w1612 w1619 w1627 w1631 w1638] -> w1594
                                frame "No rotation, No flip", Default {
                                }
                                frame "No rotation, Flip UD" {
                                w1601 = u32 0 items=["Horizontal", "Vertical", "Central", "1st Diagonal", "2nd Diagonal"] ("Type of Symmetry")
                                n522 = call "IMAQ Symmetry"("Type of Symmetry"=w1601, "Image Dst"=w1603, "Image Src"=w1603) -> ("Image Dst Out"=w1602:T4)  [unwired: 2 in, 1 out]
                                }
                                frame "No rotation, Flip LR" {
                                w1604 = u32 1 items=["Horizontal", "Vertical", "Central", "1st Diagonal", "2nd Diagonal"] ("Type of Symmetry")
                                n523 = call "IMAQ Symmetry"("Type of Symmetry"=w1604, "Image Dst"=w1606, "Image Src"=w1606) -> ("Image Dst Out"=w1605:T4)  [unwired: 2 in, 1 out]
                                }
                                frame "Clockwise, No flip" {
                                n524 = call "IMAQ Rotate"("Use Bilinear Interpolation"=FALSE, "Maintain Size"=FALSE, "Angle (degrees)"=sgl 270.0, "Image Dst"=w1609, "Image Src"=w1609) -> ("Image Dst Out"=w1607:T4)  [unwired: 5 in, 1 out]
                                }
                                frame "Clockwise, Flip UD" {
                                w1614 = u32 0 items=["Horizontal", "Vertical", "Central", "1st Diagonal", "2nd Diagonal"] ("Type of Symmetry")
                                n525 = call "IMAQ Rotate"("Use Bilinear Interpolation"=FALSE, "Maintain Size"=FALSE, "Angle (degrees)"=sgl 270.0, "Image Dst"=w1616, "Image Src"=w1616) -> ("Image Dst Out"=w1613:T4)  [unwired: 5 in, 1 out]
                                n526 = call "IMAQ Symmetry"("Type of Symmetry"=w1614, "Image Dst"=w1613, "Image Src"=w1613) -> ("Image Dst Out"=w1612:T4)  [unwired: 2 in, 1 out]
                                }
                                frame "Clockwise, Flip LR" {
                                w1621 = u32 1 items=["Horizontal", "Vertical", "Central", "1st Diagonal", "2nd Diagonal"] ("Type of Symmetry")
                                n527 = call "IMAQ Rotate"("Use Bilinear Interpolation"=FALSE, "Maintain Size"=FALSE, "Angle (degrees)"=sgl 270.0, "Image Dst"=w1623, "Image Src"=w1623) -> ("Image Dst Out"=w1620:T4)  [unwired: 5 in, 1 out]
                                n528 = call "IMAQ Symmetry"("Type of Symmetry"=w1621, "Image Dst"=w1620, "Image Src"=w1620) -> ("Image Dst Out"=w1619:T4)  [unwired: 2 in, 1 out]
                                }
                                frame "Anticlockwise, No flip" {
                                n529 = call "IMAQ Rotate"("Use Bilinear Interpolation"=FALSE, "Maintain Size"=FALSE, "Angle (degrees)"=sgl 90.0, "Image Dst"=w1626, "Image Src"=w1626) -> ("Image Dst Out"=w1627:T4)  [unwired: 5 in, 1 out]
                                }
                                frame "Anticlockwise, Flip UD" {
                                w1633 = u32 0 items=["Horizontal", "Vertical", "Central", "1st Diagonal", "2nd Diagonal"] ("Type of Symmetry")
                                n530 = call "IMAQ Rotate"("Use Bilinear Interpolation"=FALSE, "Maintain Size"=FALSE, "Angle (degrees)"=sgl 90.0, "Image Dst"=w1635, "Image Src"=w1635) -> ("Image Dst Out"=w1632:T4)  [unwired: 5 in, 1 out]
                                n531 = call "IMAQ Symmetry"("Type of Symmetry"=w1633, "Image Dst"=w1632, "Image Src"=w1632) -> ("Image Dst Out"=w1631:T4)  [unwired: 2 in, 1 out]
                                }
                                frame "Anticlockwise, Flip LR" {
                                w1640 = u32 1 items=["Horizontal", "Vertical", "Central", "1st Diagonal", "2nd Diagonal"] ("Type of Symmetry")
                                n532 = call "IMAQ Rotate"("Use Bilinear Interpolation"=FALSE, "Maintain Size"=FALSE, "Angle (degrees)"=sgl 90.0, "Image Dst"=w1642, "Image Src"=w1642) -> ("Image Dst Out"=w1639:T4)  [unwired: 5 in, 1 out]
                                n533 = call "IMAQ Symmetry"("Type of Symmetry"=w1640, "Image Dst"=w1639, "Image Src"=w1639) -> ("Image Dst Out"=w1638:T4)  [unwired: 2 in, 1 out]
                                }
                                }
                                n534 = for {
                                tunnel: w1594 -> [w1597]
                                tunnel: w1592 -> [w1596] mode=indexing
                                tunnel: w1591 -> [w1595] mode=indexing
                                n535 = case shown="\"Camera 1\"" w1596 {
                                tunnel: w1597 -> [_ w1599]
                                tunnel: w1595 -> [_ w1598]
                                frame "None", Default {
                                }
                                frame "Camera 1" {
                                n536 = call "IMAQ Copy"("Image Dst"=w1598, "Image Src"=w1599) -> ()  [unwired: 4 in, 2 out]
                                }
                                }
                                }
                                }
                                frame 1 {
                                n537 = case shown="\"Anticlockwise, Flip UD\"" w1645 {
                                tunnel: w1646 -> [w1651 w1654 w1657 w1660 w1667 w1674 w1677 w1686 w1693]
                                tunnel: [w1651 w1653 w1656 w1658 w1663 w1670 w1678 w1682 w1689] -> w1647
                                frame "No rotation, No flip", Default {
                                }
                                frame "No rotation, Flip UD" {
                                w1652 = u32 0 items=["Horizontal", "Vertical", "Central", "1st Diagonal", "2nd Diagonal"] ("Type of Symmetry")
                                n538 = call "IMAQ Symmetry"("Type of Symmetry"=w1652, "Image Dst"=w1654, "Image Src"=w1654) -> ("Image Dst Out"=w1653:T4)  [unwired: 2 in, 1 out]
                                }
                                frame "No rotation, Flip LR" {
                                w1655 = u32 1 items=["Horizontal", "Vertical", "Central", "1st Diagonal", "2nd Diagonal"] ("Type of Symmetry")
                                n539 = call "IMAQ Symmetry"("Type of Symmetry"=w1655, "Image Dst"=w1657, "Image Src"=w1657) -> ("Image Dst Out"=w1656:T4)  [unwired: 2 in, 1 out]
                                }
                                frame "Clockwise, No flip" {
                                n540 = call "IMAQ Rotate"("Use Bilinear Interpolation"=FALSE, "Maintain Size"=FALSE, "Angle (degrees)"=sgl 270.0, "Image Dst"=w1660, "Image Src"=w1660) -> ("Image Dst Out"=w1658:T4)  [unwired: 5 in, 1 out]
                                }
                                frame "Clockwise, Flip UD" {
                                w1665 = u32 0 items=["Horizontal", "Vertical", "Central", "1st Diagonal", "2nd Diagonal"] ("Type of Symmetry")
                                n541 = call "IMAQ Rotate"("Use Bilinear Interpolation"=FALSE, "Maintain Size"=FALSE, "Angle (degrees)"=sgl 270.0, "Image Dst"=w1667, "Image Src"=w1667) -> ("Image Dst Out"=w1664:T4)  [unwired: 5 in, 1 out]
                                n542 = call "IMAQ Symmetry"("Type of Symmetry"=w1665, "Image Dst"=w1664, "Image Src"=w1664) -> ("Image Dst Out"=w1663:T4)  [unwired: 2 in, 1 out]
                                }
                                frame "Clockwise, Flip LR" {
                                w1672 = u32 1 items=["Horizontal", "Vertical", "Central", "1st Diagonal", "2nd Diagonal"] ("Type of Symmetry")
                                n543 = call "IMAQ Rotate"("Use Bilinear Interpolation"=FALSE, "Maintain Size"=FALSE, "Angle (degrees)"=sgl 270.0, "Image Dst"=w1674, "Image Src"=w1674) -> ("Image Dst Out"=w1671:T4)  [unwired: 5 in, 1 out]
                                n544 = call "IMAQ Symmetry"("Type of Symmetry"=w1672, "Image Dst"=w1671, "Image Src"=w1671) -> ("Image Dst Out"=w1670:T4)  [unwired: 2 in, 1 out]
                                }
                                frame "Anticlockwise, No flip" {
                                n545 = call "IMAQ Rotate"("Use Bilinear Interpolation"=FALSE, "Maintain Size"=FALSE, "Angle (degrees)"=sgl 90.0, "Image Dst"=w1677, "Image Src"=w1677) -> ("Image Dst Out"=w1678:T4)  [unwired: 5 in, 1 out]
                                }
                                frame "Anticlockwise, Flip UD" {
                                w1684 = u32 0 items=["Horizontal", "Vertical", "Central", "1st Diagonal", "2nd Diagonal"] ("Type of Symmetry")
                                n546 = call "IMAQ Rotate"("Use Bilinear Interpolation"=FALSE, "Maintain Size"=FALSE, "Angle (degrees)"=sgl 90.0, "Image Dst"=w1686, "Image Src"=w1686) -> ("Image Dst Out"=w1683:T4)  [unwired: 5 in, 1 out]
                                n547 = call "IMAQ Symmetry"("Type of Symmetry"=w1684, "Image Dst"=w1683, "Image Src"=w1683) -> ("Image Dst Out"=w1682:T4)  [unwired: 2 in, 1 out]
                                }
                                frame "Anticlockwise, Flip LR" {
                                w1691 = u32 1 items=["Horizontal", "Vertical", "Central", "1st Diagonal", "2nd Diagonal"] ("Type of Symmetry")
                                n548 = call "IMAQ Rotate"("Use Bilinear Interpolation"=FALSE, "Maintain Size"=FALSE, "Angle (degrees)"=sgl 90.0, "Image Dst"=w1693, "Image Src"=w1693) -> ("Image Dst Out"=w1690:T4)  [unwired: 5 in, 1 out]
                                n549 = call "IMAQ Symmetry"("Type of Symmetry"=w1691, "Image Dst"=w1690, "Image Src"=w1690) -> ("Image Dst Out"=w1689:T4)  [unwired: 2 in, 1 out]
                                }
                                }
                                n550 = call "IMAQ Copy"("Image Dst"=w1650, "Image Src"=w1647) -> ("Image Dst Out"=w1648:T4)  [unwired: 4 in, 1 out]
                                n551 = property class="ImageControl"(reference=w1649, "Value"=w1648) -> ()  [unwired: 1 in, 2 out]
                                }
                                }
                              }
                              frame True {
                              }
                            }
                            n552 = property class="Bool (strict)"(reference=w1495) -> ("Value"=w1498:bool)  [unwired: 1 in, 2 out]
                            n553 = Not(x=w1498) -> (.not. x?=w1497:bool)
                          }
                        }
                      }
                    }
                    frame True {
                    }
                  }
                }
                frame #1 {
                  n554 = Send Notification(notification=TRUE, notifier=w1697) -> ()  [unwired: 1 in, 2 out]
                }
              }
              n555 = node-c288(w734, 10 ("Priority")) -> (w755:T13)  [unwired: 2 in]
              n556 = timed-loop {
                timing: w755 -> [_]
                timing-out: [_] -> w754
                tunnel: w753 -> [w776]
                tunnel: w749 -> [w774]
                tunnel: w747 -> [w773]
                tunnel: w746 -> [_]
                stop <- w775 stop-if-true
                n557 = node-c288() -> ()  [unwired: 1 in, 1 out]
                n558 = Get Notifier Status(notifier=w776) -> (current notification=w775:bool)  [unwired: 1 in, 4 out]
                n559 = Unbundle By Name(w774) -> ("Offset and gain"=w769:dbl[][], "RGB Channels"=w772:T19, "RGB buffers"=w771:T4[], "Current camera"=w770:i32)
                n560 = case shown="0" w770 {
                  tunnel: w769 -> [_ w803]
                  tunnel: w772 -> [_ w802]
                  tunnel: w771 -> [_ w777]
                  tunnel: w773 -> [_ w799]
                  frame 1, Default {
                  }
                  frame 0 {
                    w787 = 0 ("X Resolution")
                    w790 = u16 0 items=["RGB", "HSL", "HSV", "HSI"] ("Color Mode")
                    n561 = Index Array(array=w777, index #1=0 ("index"), index #2=1 ("index")) -> (element #1=w784:T4, element #2=w797:T4)
                    n562 = Array Subset(array=w777, index=2 ("length"), length=3 ("index")) -> (w801:T4[])
                    n563 = Array Subset(array=w777, index=5 ("length"), length=3 ("index")) -> (w778:T4[])
                    n564 = for {
                      tunnel: w801 -> [w817] mode=indexing
                      tunnel: w803 -> [w816] mode=indexing
                      tunnel: w802 -> [w818] mode=indexing
                      tunnel: [w815] -> w796 mode=indexing
                      tunnel: w797 -> [w814]
                      shift-right: [w810] -> w786
                      shift-left: w787 -> [w813]
                      shift-right: [w811] -> w785
                      shift-left: w787 -> [w812]
                      tunnel: w784 -> [w809]
                      tunnel: w778 -> [w808] mode=indexing
                      n565 = case shown="\"Camera 1\", Default" w818 {
                        tunnel: w817 -> [w822 w839]
                        tunnel: w816 -> [_ w849]
                        tunnel: [w828 w838] -> w815
                        tunnel: w814 -> [_ w851]
                        tunnel: w813 -> [w826 w835]
                        tunnel: w812 -> [w824 w833]
                        tunnel: [w824 w832] -> w811
                        tunnel: [w826 w831] -> w810
                        tunnel: w809 -> [w827 _]
                        tunnel: w808 -> [_ w830]
                        frame "None" {
                          n566 = call "IMAQ GetImageSize"("Image"=w827) -> ("Y Resolution"=w823:i32, "X Resolution"=w825:i32)  [unwired: 3 in, 1 out]
                          n567 = Max & Min(x=w826, y=w825) -> (max(x,y)=w820:i32)  [unwired: 1 out]
                          n568 = Max & Min(x=w824, y=w823) -> (max(x,y)=w819:i32)  [unwired: 1 out]
                          n569 = call "IMAQ SetImageSize"("Y Resolution"=w819, "X Resolution"=w820, "Image"=w822) -> ("Image Out"=w821:T4)  [unwired: 2 in, 1 out]
                          n570 = call "IMAQ FillImage"("Pixel Value (U8, U16, I16, Float)"=sgl 0.0, "Image"=w821) -> ("Image Out"=w828:T4)  [unwired: 8 in, 1 out]
                        }
                        frame "Camera 1", Default {
                          w840 = T17 0 items=["Grayscale (U8)", "Grayscale (I16)", "Grayscale (SGL)", "Complex (CSG)", "RGB (U32)", "HSL (U32)", "RGB (U64)", "Grayscale (U16)"] ("Image Type")
                          w850 = T17 2 items=["Grayscale (U8)", "Grayscale (I16)", "Grayscale (SGL)", "Complex (CSG)", "RGB (U32)", "HSL (U32)", "RGB (U64)", "Grayscale (U16)"] ("Image Type")
                          n571 = call "IMAQ GetImageSize"("Image"=w830) -> ("Y Resolution"=w834:i32, "X Resolution"=w836:i32, "error out"=w837:errorcluster)  [unwired: 3 in]
                          n572 = Index Array(array=w849, index #1=0 ("index"), index #2=1 ("index")) -> (element #1=w846:dbl, element #2=w842:dbl)
                          n573 = call "IMAQ Cast Image"("Image Type"=w850, "error in (no error)"=w837, "Image Dst"=w851, "Image Src"=w830) -> ("Image Dst Out"=w845:T4)  [unwired: 6 in, 1 out]
                          n574 = Max & Min(x=w835, y=w836) -> (max(x,y)=w831:i32)  [unwired: 1 out]
                          n575 = Max & Min(x=w833, y=w834) -> (max(x,y)=w832:i32)  [unwired: 1 out]
                          n576 = call "IMAQ Add"("Image Src A"=w845, "Constant"=w846, "Image Dst"=w845) -> ("Image Dst Out"=w843:T4, "error out"=w844:errorcluster)  [unwired: 4 in]
                          n577 = call "IMAQ Multiply"("Image Src A"=w843, "Constant"=w842, "Image Dst"=w843, "error in (no error)"=w844) -> ("Image Dst Out"=w841:T4)  [unwired: 3 in, 1 out]
                          n578 = call "IMAQ Cast Image"("Image Type"=w840, "Image Dst"=w839, "Image Src"=w841) -> ("Image Dst Out"=w838:T4)  [unwired: 7 in, 1 out]
                        }
                      }
                    }
                    n579 = Index Array(array=w796, index #1=0 ("index"), index #2=1 ("index"), index #3=2 ("index")) -> (element #1=w788:T4, element #2=w792:T4, element #3=w791:T4)
                    n580 = call "IMAQ SetImageSize"("Y Resolution"=w785, "X Resolution"=w786, "Image"=w784) -> ("error out"=w782:errorcluster, "Image Out"=w789:T4)  [unwired: 2 in]
                    n581 = call "IMAQ ReplaceColorPlane"("Image Src"=w789, "Color Mode"=w790, "Image Dst"=w789, "Red or Hue Plane"=w788, "Green or Sat Plane"=w792, "error in (no error)"=w782, "Blue or Luma or Val or Inten Plane"=w791) -> ("Image Dst Out"=w783:T4, "error out"=w781:errorcluster)  [unwired: 7 in]
                    n582 = case shown="No Error" w781 {
                      tunnel: w799 -> [w807 _]
                      tunnel: w783 -> [w806 _]
                      frame No Error {
                        n583 = property class="ImageControl"(reference=w807, "Value"=w806) -> ()  [unwired: 1 in, 2 out]
                      }
                      frame Error {
                      }
                    }
                  }
                }
                n584 = node-c288() -> ()  [unwired: 1 in, 1 out]
              }
              n585 = node-c288(w754) -> ()  [unwired: 1 out]
            }
            frame #3 {
              n586 = disable-structure shown="Enabled" {
                disable-tunnel: w1705 -> [_ w1757]
                frame Disabled {
                }
                frame Enabled {
                  n587 = for {
                    tunnel: w1757 -> [w1759] mode=indexing
                    n588 = call <vilib>:"IMAQdx Stop Acquisition.vi"("Session In"=w1759) -> ("Session Out"=w1758:T3)  [unwired: 9 in, 1 out]
                    n589 = call <vilib>:"IMAQdx Unconfigure Acquisition.vi"("Session In"=w1758) -> ()  [unwired: 9 in, 2 out]
                  }
                }
              }
              n590 = case shown="\"'tiff'\", \"tif\"" w1704 {
                tunnel: w1703 -> [_ _ w1747]
                tunnel: w1702 -> [w1708 _ _]
                tunnel: w1701 -> [w1724 _ _]
                tunnel: w1700 -> [w1712 _ w1739]
                tunnel: w1699 -> [w1719 _ w1746]
                tunnel: w1698 -> [w1718 _ _]
                frame "'tiff'", "tif" {
                  n591 = Dequeue Element(queue=w1708) -> (queue out=w1706:refnum<queue>, element=w1707:T11)  [unwired: 2 in, 2 out]
                  n592 = Flush Queue(queue=w1712) -> (queue out=w1716:refnum<queue>, remaining elements=w1715:T25, error out=w1714:errorcluster)  [unwired: 1 in]
                  n593 = Preview Queue Element(queue=w1718) -> (element=w1717:u32[])  [unwired: 2 in, 3 out]
                  n594 = call "TIFFStream Close.vi"("Current and next IFD offset"=w1717, "Image data reference"=w1724, "File data"=w1707) -> ()  [unwired: 8 in, 1 out]
                  n595 = Release Queue(queue=w1706) -> ()  [unwired: 2 in, 3 out]
                  n596 = for {
                    tunnel: w1715 -> [w1733] mode=indexing
                    tunnel: [w1732] -> w1713 mode=indexing
                    n597 = Unbundle(w1733) -> ("Camera identity"=w1730:enum16{"Camera 1", "Camera 2", "Camera 3"}, "Timestamp"=w1731:u64)
                    n598 = Increment(x=w1730) -> (x+1=w1725:enum16{"Camera 1", "Camera 2", "Camera 3"})
                    n599 = Number To Decimal String(number=w1731) -> (decimal integer string=w1728:string)  [unwired: 1 in]
                    n600 = Number To Decimal String(number=w1725) -> (decimal integer string=w1729:string)  [unwired: 1 in]
                    n601 = call <vilib>:"Space Constant.vi"() -> ("String"=w1727:string)
                    n602 = Concatenate Strings(w1729, w1727, w1728, "\r") -> (w1732:string)
                  }
                  n603 = Release Queue(queue=w1716, error in (no error)=w1714) -> ()  [unwired: 1 in, 3 out]
                  n604 = Strip Path(path=w1719) -> (stripped path=w1723:path)  [unwired: 1 out]
                  n605 = call <vilib>:"Get File Extension.vi"("file"=w1719) -> ("filename without extension"=w1721:string)  [unwired: 6 in, 4 out]
                  n606 = Concatenate Strings(w1721, "_FrameOrder.txt" ("string")) -> (w1722:string)
                  n607 = Build Path(base path=w1723, name or relative path=w1722) -> (appended path=w1711:path)
                  n608 = Concatenate Strings(w1713) -> (w1710:string)
                  n609 = Write to Text File(file (use dialog)=w1711, text=w1710) -> (refnum out=w1709:refnum<file>)  [unwired: 2 in, 2 out]
                  n610 = Close File(refnum=w1709) -> ()  [unwired: 1 in, 2 out]
                }
                frame "None", Default {
                }
                frame "dat", "u16" {
                  n611 = Close File(refnum=w1747) -> ()  [unwired: 1 in, 2 out]
                  n612 = Flush Queue(queue=w1739) -> (queue out=w1740:refnum<queue>, remaining elements=w1735:T25, error out=w1738:errorcluster)  [unwired: 1 in]
                  n613 = Strip Path(path=w1746) -> (stripped path=w1745:path)  [unwired: 1 out]
                  n614 = call <vilib>:"Get File Extension.vi"("file"=w1746) -> ("filename without extension"=w1743:string)  [unwired: 6 in, 4 out]
                  n615 = Concatenate Strings(w1743, "_FrameOrder.txt" ("string")) -> (w1744:string)
                  n616 = Release Queue(queue=w1740, error in (no error)=w1738) -> ()  [unwired: 1 in, 3 out]
                  n617 = for {
                    tunnel: w1735 -> [w1756] mode=indexing
                    tunnel: [w1755] -> w1736 mode=indexing
                    n618 = Unbundle(w1756) -> ("Camera identity"=w1753:enum16{"Camera 1", "Camera 2", "Camera 3"}, "Timestamp"=w1754:u64)
                    n619 = Increment(x=w1753) -> (x+1=w1748:enum16{"Camera 1", "Camera 2", "Camera 3"})
                    n620 = Number To Decimal String(number=w1754) -> (decimal integer string=w1751:string)  [unwired: 1 in]
                    n621 = Number To Decimal String(number=w1748) -> (decimal integer string=w1752:string)  [unwired: 1 in]
                    n622 = call <vilib>:"Space Constant.vi"() -> ("String"=w1750:string)
                    n623 = Concatenate Strings(w1752, w1750, w1751, "\r") -> (w1755:string)
                  }
                  n624 = Build Path(base path=w1745, name or relative path=w1744) -> (appended path=w1741:path)
                  n625 = Concatenate Strings(w1736) -> (w1734:string)
                  n626 = Write to Text File(file (use dialog)=w1741, text=w1734) -> (refnum out=w1737:refnum<file>)  [unwired: 2 in, 2 out]
                  n627 = Close File(refnum=w1737) -> ()  [unwired: 1 in, 2 out]
                }
              }
            }
          }
        }
      }
    }
    frame "Get status" {
      n628 = Variant To Data(type=w1769, Variant=w1770) -> (data=w1768:T6)  [unwired: 1 in, 1 out]
      n629 = Unbundle By Name(w1768) -> ("Camera References"=w1767:T3[], "Current camera"=w1766:i32)
      n630 = Decrement(x=w1766) -> (x-1=w1762:i32)
      n631 = Max & Min(x=w1762, y=1) -> (max(x,y)=w1760:i32)  [unwired: 1 out]
      n632 = Index Array(array=w1767, index=w1760) -> (element=w1765:T3)
      n633 = property class="IMAQdx"(reference=w1765, "ActiveAttribute"="CameraAttributes::DeviceControl::DeviceTemperature") -> (error out=w1764:errorcluster, "ValueDBL"=w1771:dbl)  [unwired: 1 in, 1 out]
      n634 = Unbundle By Name(w1764) -> ("status"=w1763:bool)
      n635 = Bundle By Name(cluster=w1774, "System OK?"=w1763, "Temperature"=w1771) -> (w1773:T1)
    }
    frame "Other settings" {
      n636 = Variant To Data(type=w1790, Variant=w1791) -> (data=w1786:T6)  [unwired: 1 in, 1 out]
      n637 = Unbundle By Name(w1786) -> ("Offset and gain"=w1777:dbl[][], "Camera References"=w1789:T3[], "Current camera"=w1788:i32, "Which cameras record"=w1787:bool[], "RGB Channels"=w1779:T19, "Image buffers"=w1778:T4[], "Camera orientation"=w1776:T18)
      n638 = call "PointGrey Grasshopper_Settings.vi"("Camera References"=w1789, "Offset and gain"=w1777, "Camera to address"=w1788, "Camera orientation"=w1776, "Which cameras record"=w1787, "RGB Channels in"=w1779, "Image buffers"=w1778) -> ("Offset gain out"=w1781:dbl[][], "Camera to address out"=w1782:i32, "Camera orientation out"=w1775:T18, "Which cameras record out"=w1785:bool[], "RGB Channels out"=w1780:T19)  [unwired: 4 in]
      n639 = Bundle By Name(cluster=w1786, "Offset and gain"=w1781, "Current camera"=w1782, "Which cameras record"=w1785, "RGB Channels"=w1780, "Camera orientation"=w1775) -> (w1783:T6)
      n640 = To Variant(anything=w1783) -> (Variant=w1784:variant)
    }
  }
  "Status" <- w8
  "Camera-specific out" <- w5
